vi "MC_10_19a_JW1.vi"() -> ()   [LabVIEW 2011]
uses:
  <vilib>/Utility/file.llb/Read From Spreadsheet File (string).vi
  <vilib>/Utility/inputDevices.llb/keyboardAcquire.vi
  <vilib>/Utility/file.llb/Write To Spreadsheet File (string).vi
  <vilib>/regexp/Match Regular Expression.xnode
panel:
  out "Column":string
  out "Row":string
  out "Date Recorded":string="Date Recorded"
  out "Concentration Recorded":string
  out "Solvent Recorded":string
  out "Method Recorded":string
  in  "?":T1(tab)
  out "Material Recorded":string
  in  "Treatment Concentration (mM):":dbl
  in  "Surface Treatment:":string
  in  "# Drops:":dbl
  in  "Solution Temp (C):":dbl
  in  "Relative Humidity (%):":dbl
  in  "Room Temp (F):":dbl
  in  "Time (s):":dbl
  out "Accel (RPM/s):":dbl
  in  "RPM:":dbl
  in  "Wait Time (s):":dbl
  in  "Sample #:":dbl
  in  "Fabricator:":string
  in  "Data File":path
  out "Data Folder":path
  in  "Image Folder":path
  out "Image File":path
  in  "Ramp (s):":dbl
  out "Mobility":dbl format="%#_4e"
  out "Length":dbl
  out "Width":dbl
  out "Dielectric (d)":dbl
  out "XY Graph":cluster{dbl[], dbl[]}[](graph)
  in  "NumPts":dbl=5.0
  in  "Cancel Button":bool
  in  "Next Button":bool
  in  "Previous Button":bool
  in  "Up Button":bool
  in  "Down Button":bool
  out "Data Name":string
  in  "Save Changes?":bool
  in  "New Dielectric":dbl
  in  "New Length":dbl
  in  "New Width":dbl
  out "New Mobility":dbl format="%#_4e"
  in  "Slide":dbl(slide) step=1.0 scale=-14.3..84.0 scale format="%#_1p"
  in  "Blank Button":bool
  in  "Zoom":i16(slide)=-3 scale=-5.0..5.0
  out "Image Out 2":T2(plugin-control)
  out "Image Out":T2(plugin-control)
  in  "Magnification":u16(ring) items=["5x", "10x", "20x", "50x", "80x"]
  out "Total Width":dbl
  out "Distances":dbl[](array[numeric])
  in  "Undo Button":bool
  in  "Remove Button":bool
  out "Recorded Mobility":dbl format="%#_4e"
  out "Index 3":string
  out "Image Name":string
  in  "Export":bool
  out "Threshold V":dbl
  out "New Vt":dbl
  in  "Manual":bool
  out "XY Graph 2":cluster{dbl[], dbl[]}[](graph)
  in  "Next Button 2":bool
  in  "Previous Button 2":bool
  in  "Slide 2":dbl(slide) step=1.0 scale=-1.0..82.0 scale format="%#_1p"
  out "S.T.S.":dbl
  out "New S.T.S.":dbl
  in  "NumPts 2":dbl=5.0
  out "Vt recorded":dbl
  out "STS recorded":dbl
  out "On/Off":dbl format="%#_3e"
  in  "Save Changes? 2":bool
  in  "Save Changes? 3":bool
  out "Export \nHeaders":string[](array[string])
  out "Current\nRecord":string[](array[string])
  out "Full Database":string[][](array[string])
  out "String":string
  in  "No Image":path=path "C:/Program Files/Mega Awesome/Image Not Found.png"
  in  "Project":path=path "C:/Program Files/Mega Awesome/DeviceData.opj"
  out "Index 2":dbl
  out "Array 8":dbl[](array[numeric])
  out "Array 7":dbl[](array[numeric])
  out "ROI Descriptor out":T3 {"Contours"."Type" items=["No Selection", "Point", "Line", "Rectangle", "Oval", "Polygon", "Freehand Region", "Annulus", "Unused2", "Unused3", "Broken Line", "Freehand Line", "Rotated Rectangle"]}
  out "ROI Descriptor":T3 {"Contours"."Type" items=["No Selection", "Point", "Line", "Rectangle", "Oval", "Polygon", "Freehand Region", "Annulus", "Unused2", "Unused3", "Broken Line", "Freehand Line", "Rotated Rectangle"]}
  out "Numeric 3":dbl
  out "Array 6":dbl[][](array[numeric])
  out "Cluster":T4
  out "Array 5":dbl[](array[numeric])
  out "Array 4":dbl[](array[numeric])
  out "Array 3":dbl[](array[numeric])
  out "Numeric 2":dbl
  out "Numeric":dbl
  out "Array 2":dbl[](array[numeric])
  out "Array":dbl[](array[numeric])
  out "Index":dbl
  out "Table Control 2":string[][](table)
  out "Table Control":string[][](table)
  in  "Row Start":dbl=20.0
  # "Data Locations"
  # "Data Location"
  # "Image Location"
  # "Sample Properties"
  # "Recorded"
  # "Calculated"
  # "Re-Calculated"
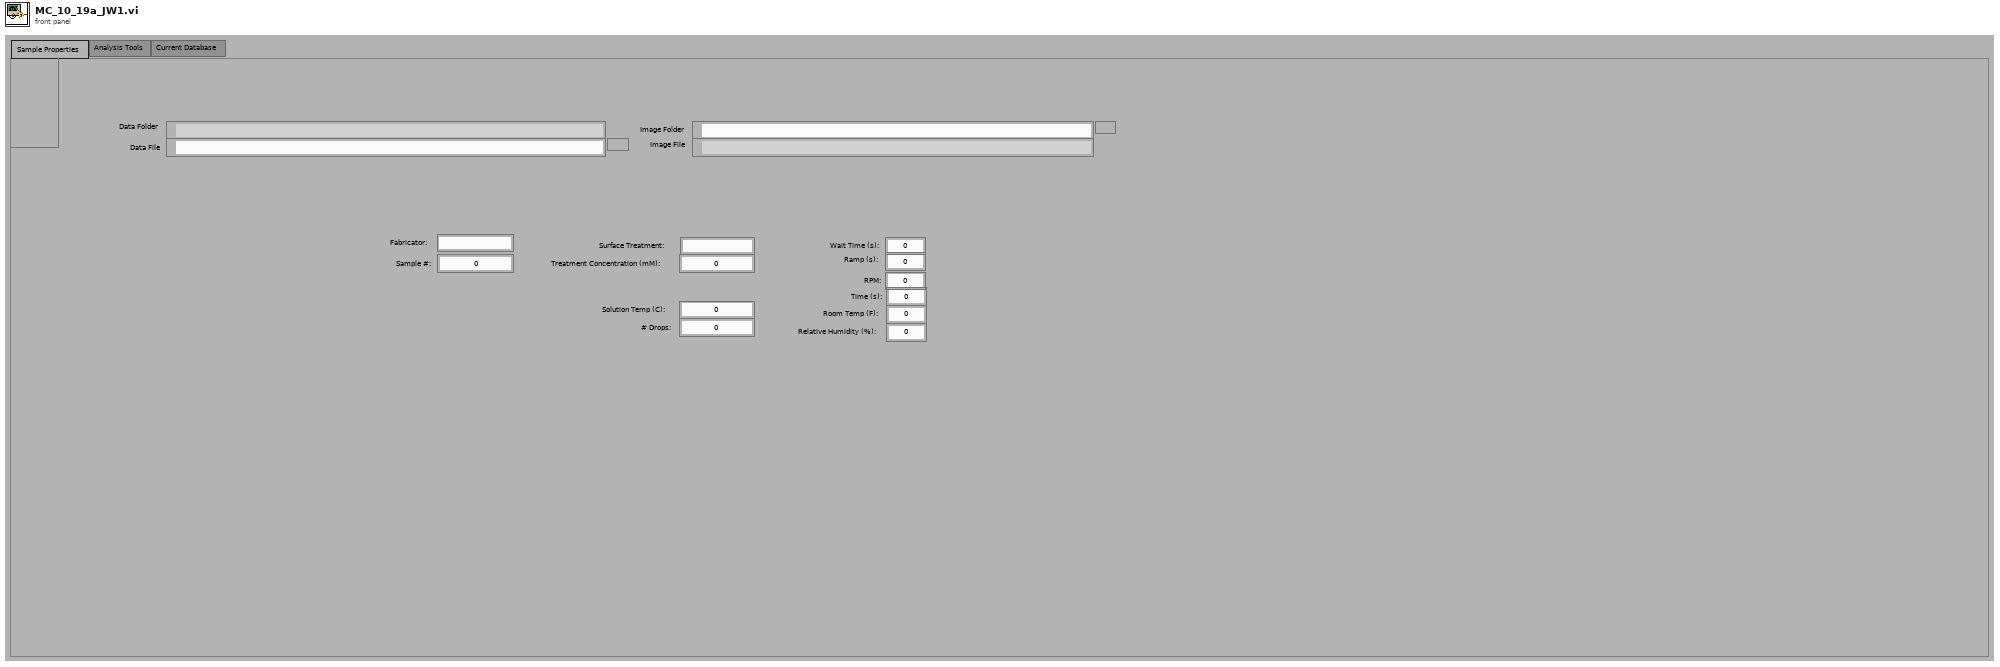
[diagram p1: front panel]
types:
  T1 = enum32{"Sample Properties", "Analysis Tools", "Current Database"}
  T2 = typedef "IMAQ Image.ctl" = refnum<image>
  T3 = typedef "ROI Descriptor" = cluster{"Global Rectangle":i32[], "Contours":cluster{"ID":enum32{"External", "Internal"}, "Type":u32, "Coordinates":i32[]}[]}
  T4 = cluster{"Numeric":dbl, "Numeric 2":dbl, "Numeric 3":dbl, "Numeric 4":dbl}
  T5 = cluster{"[0]":cluster{dbl[], dbl[]}, "[1]":cluster{dbl[], dbl[]}, "[2]":cluster{dbl[], dbl[]}, "[3]":cluster{dbl[], dbl[]}, "[4]":cluster{dbl[], dbl[]}, "[5]":cluster{dbl[], dbl[]}, "[6]":cluster{dbl[], dbl[]}, "[7]":cluster{dbl[], dbl[]}, "[8]":cluster{dbl[], dbl[]}}
  T6 = cluster{"Vt":dbl, "STS":dbl, "On/Off":dbl, "Deposition":string, "Solvent":string, "Concentration":string, "Material":string}
  T7 = cluster{"Global Rectangle":i32[], "Contours":cluster{"Contour Type":u32, "ROI Type":u32, "Points":i32[]}[]}
  T8 = typedef "LVBoundsTypeDef.ctl" = cluster{"Width":u32, "Height":u32}
  T9 = cluster{"Contour Type":u32, "ROI Type":u32, "Points":i32[]}[]
  T10 = enum16{"0", "1", "2", "3", "4", "5", "6", "7", "8", "9", "A", "B", "C", "D", "E", "F", "G", "H", "I", "J", "K", "L", "M", "N", "O", "P", "Q", "R", "S", "T", "U", "V", "W", "X", "Y", "Z", "F1", "F2", "F3", "F4", "F5", "F6", "F7", "F8", "F9", "F10", "F11", "F12", "F13", "F14", "F15", "ADD", "BACK", "BACKSLASH", "CAPITAL", "COMMA", "DECIMAL", "DELETE", "DIVIDE", "DOWN", "END", "EQUALS", "ESCAPE", "GRAVE (`)", "HOME", "INSERT", "LBRACKET", "LCONTROL", "LEFT", "L ALT", "LSHIFT", "LWIN", "MINUS", "MULTIPLY", "NEXT", "NUMLOCK", "NUMPAD_0", "NUMPAD_1", "NUMPAD_2", "NUMPAD_3", "NUMPAD_4", "NUMPAD_5", "NUMPAD_6", "NUMPAD_7", "NUMPAD_8", "NUMPAD_9", "PAUSE", "PERIOD", "PRIOR (PG UP)", "RBRACKET", "RCONTROL", "RETURN", "RIGHT", "R ALT", "RSHIFT", "RWIN", "SCROLL", "SEMICOLON", "SLASH", "SPACE", "SUBTRACT", "TAB", "UP", "ENTER (num pad)", "' (quote)"}[]
  T11 = cluster{i32[], cluster{"Contour Type":u32, "ROI Type":u32, "Points":i32[]}[]}
  T12 = enum16{"0", "1", "2", "3", "4", "5", "6", "7", "8", "9", "A", "B", "C", "D", "E", "F", "G", "H", "I", "J", "K", "L", "M", "N", "O", "P", "Q", "R", "S", "T", "U", "V", "W", "X", "Y", "Z", "F1", "F2", "F3", "F4", "F5", "F6", "F7", "F8", "F9", "F10", "F11", "F12", "F13", "F14", "F15", "ADD", "BACK", "BACKSLASH", "CAPITAL", "COMMA", "DECIMAL", "DELETE", "DIVIDE", "DOWN", "END", "EQUALS", "ESCAPE", "GRAVE (`)", "HOME", "INSERT", "LBRACKET", "LCONTROL", "LEFT", "L ALT", "LSHIFT", "LWIN", "MINUS", "MULTIPLY", "NEXT", "NUMLOCK", "NUMPAD_0", "NUMPAD_1", "NUMPAD_2", "NUMPAD_3", "NUMPAD_4", "NUMPAD_5", "NUMPAD_6", "NUMPAD_7", "NUMPAD_8", "NUMPAD_9", "PAUSE", "PERIOD", "PRIOR (PG UP)", "RBRACKET", "RCONTROL", "RETURN", "RIGHT", "R ALT", "RSHIFT", "RWIN", "SCROLL", "SEMICOLON", "SLASH", "SPACE", "SUBTRACT", "TAB", "UP", "ENTER (num pad)", "' (quote)"}
  T13 = cluster{string, sgl, bool, bool, bool, bool, bool, bool, i32}
  T14 = cluster{i32, cluster{string, sgl, bool, bool, bool, bool, bool, bool, i32}, i32, i32}
  T15 = cluster{"Contour Type":u32, "ROI Type":u32, "Points":i32[]}
  T16 = cluster{"Points[0]":i32, "Points[1]":i32, "Points[2]":i32, "Points[3]":i32, "Points[4]":i32, "Points[5]":i32, "Points[6]":i32, "Points[7]":i32, "Points[8]":i32}
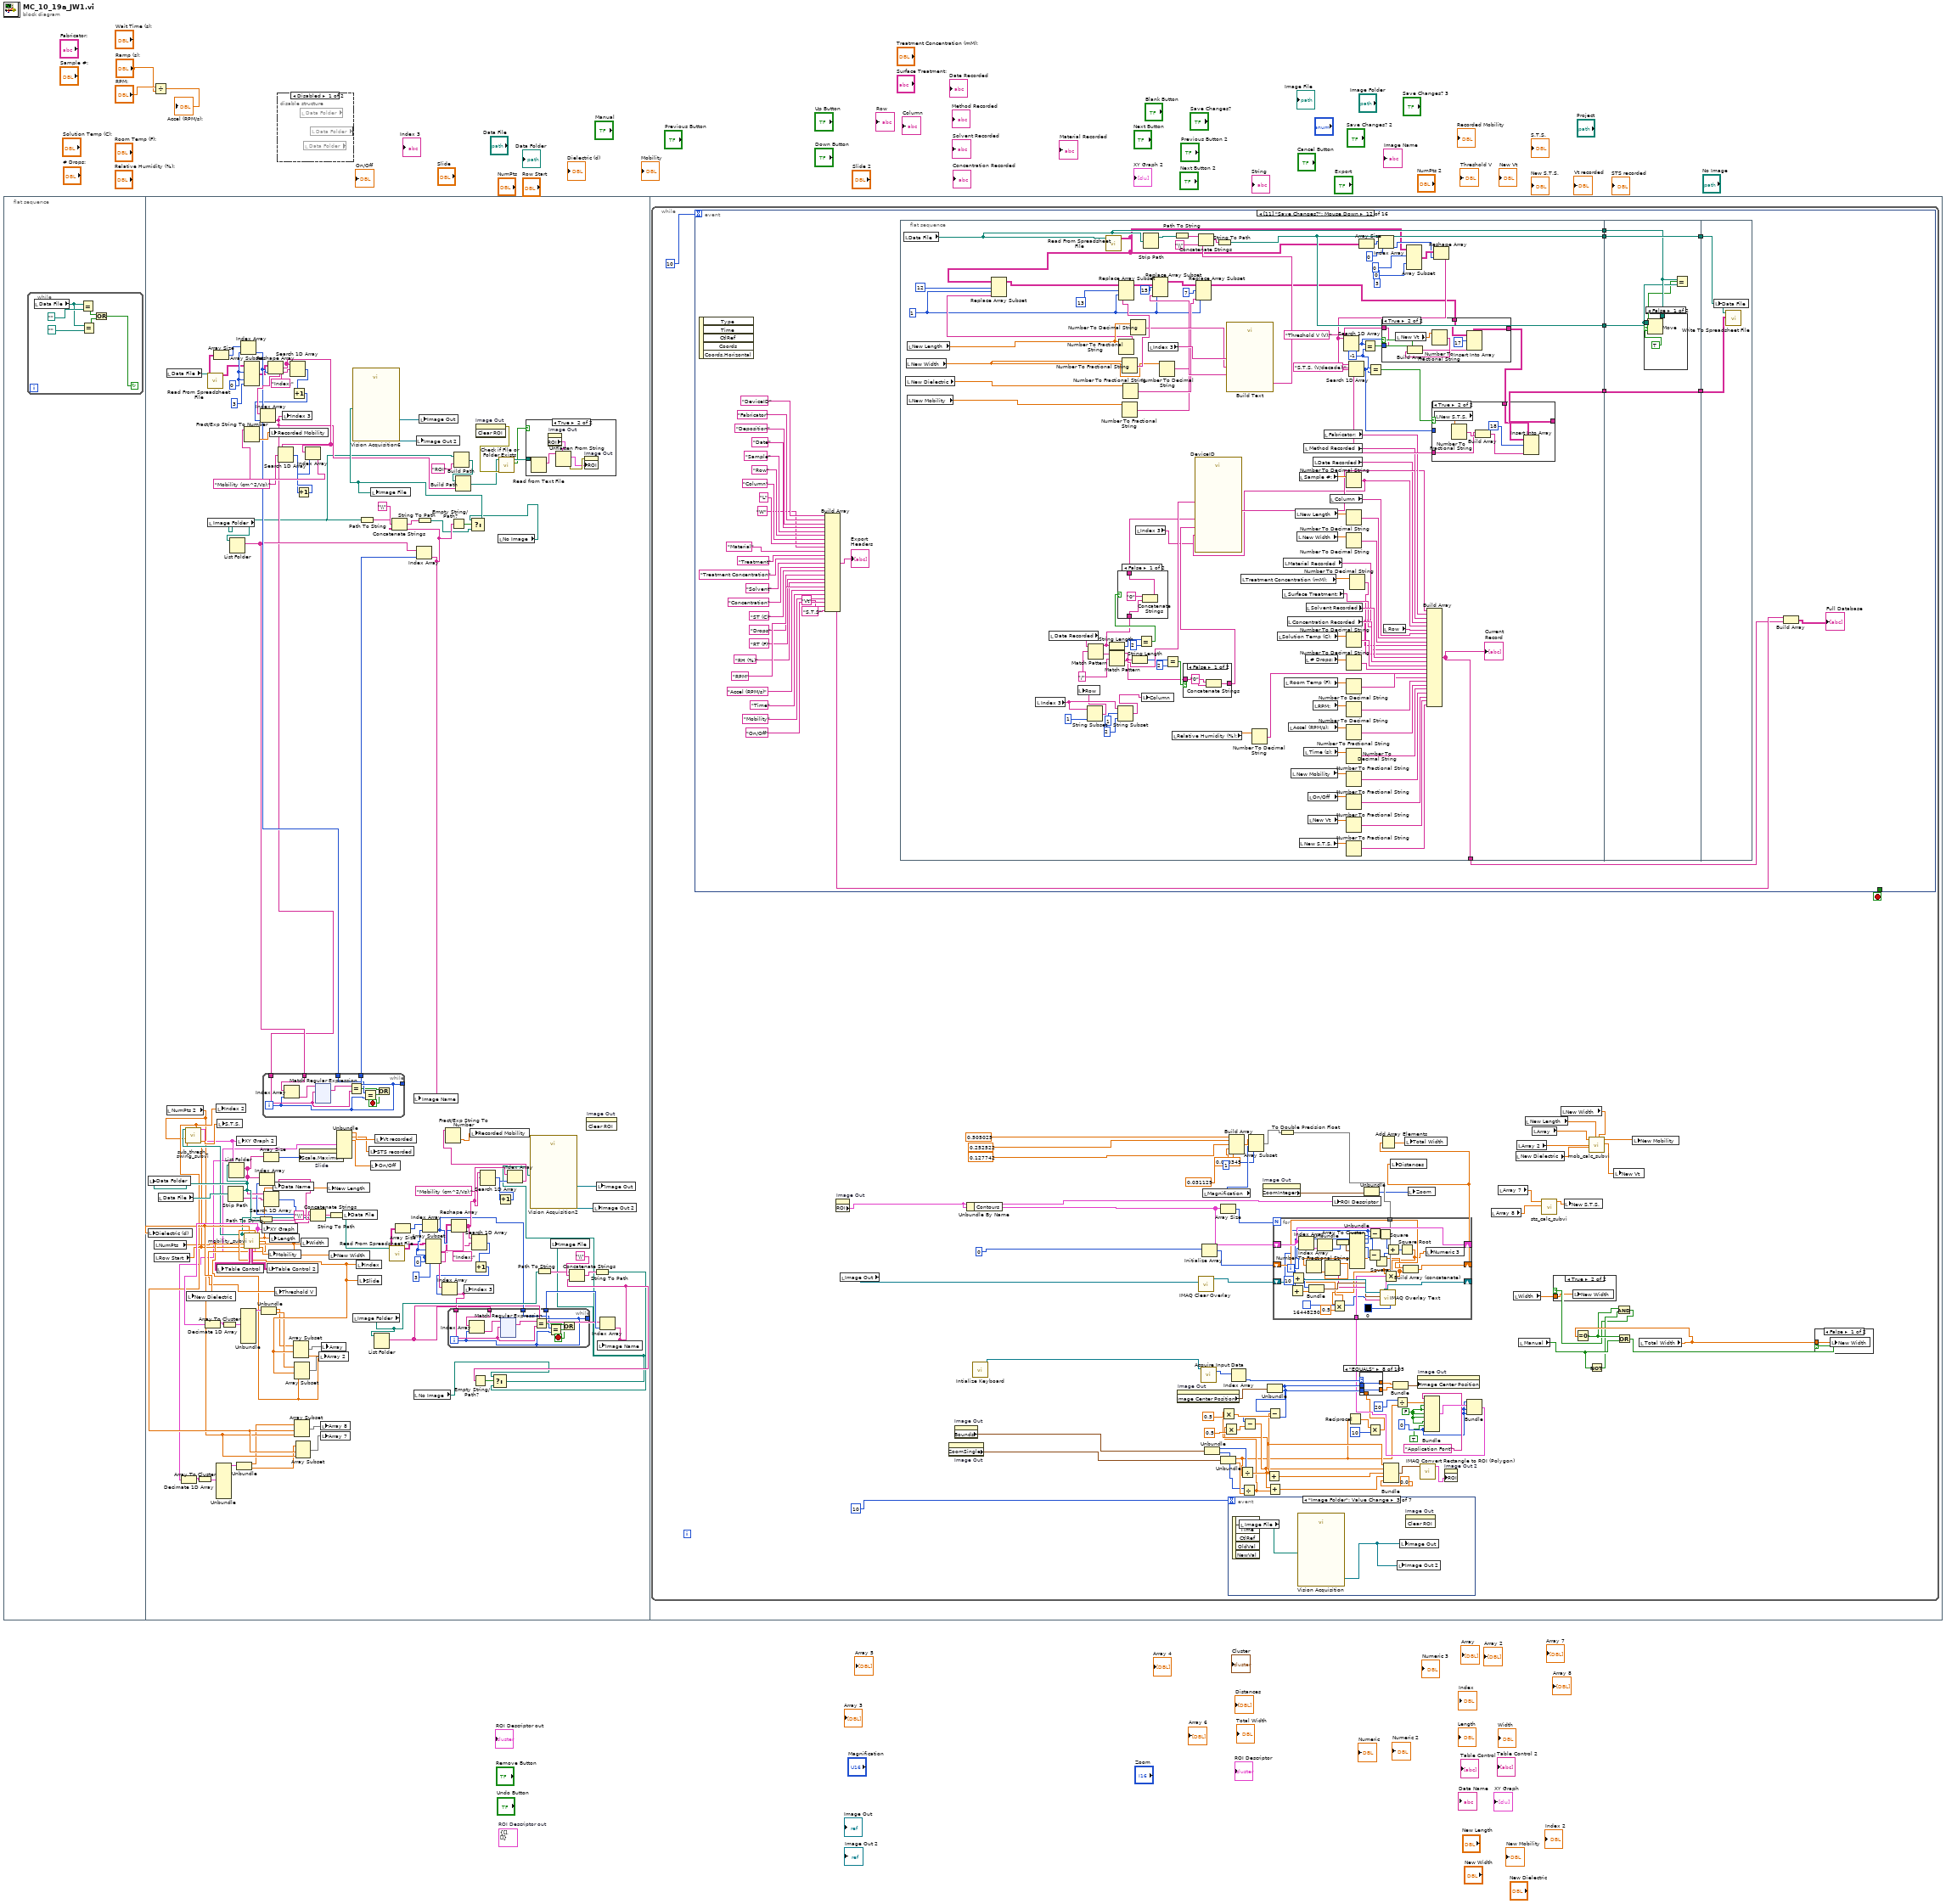
[diagram p0: block diagram]
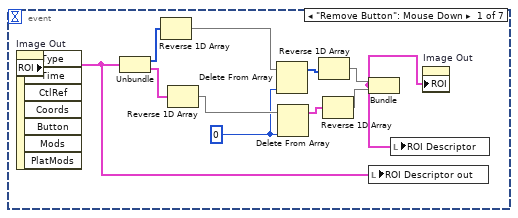
[diagram p5: hidden frame]
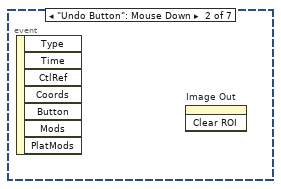
[diagram p6: hidden frame]
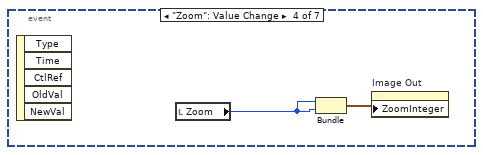
[diagram p7: hidden frame]
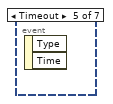
[diagram p8: hidden frame]
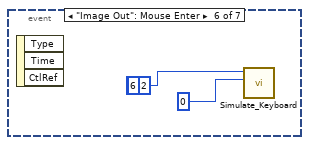
[diagram p9: hidden frame]
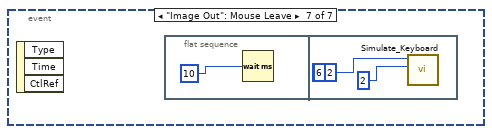
[diagram p10: hidden frame]
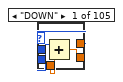
[diagram p11: hidden frame]
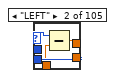
[diagram p12: hidden frame]
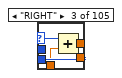
[diagram p13: hidden frame]
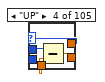
[diagram p14: hidden frame]
diagram:
  (unwired) T3 {"Global Rectangle"=[], "Contours"=[]}  # ROI Descriptor out
  n1 = flat-sequence {
    frame #0 {
      n2 = while {
        stop <- w4 continue-if-true
        n3 = local read "Data File"() -> (w6:path)
        n4 = Equal?(x=w6, y=path "") -> (x = y?=w8:bool)
        n5 = Equal?(x=w6, y=path "") -> (x = y?=w7:bool)
        n6 = Or(x=w8, y=w7) -> (x .or. y?=w4:bool)
      }
    }
    frame #1 {
      w70 = 0
      w100 = 0
      n7 = local read "NumPts"() -> (w45:dbl)
      n8 = local read "Row Start"() -> (w44:dbl)
      n9 = local read "Data File"() -> (w74:path)
      n10 = local read "Data File"() -> (w95:path)
      n11 = local read "NumPts 2"() -> (w39:dbl)
      n12 = call-poly <vilib>:"Read From Spreadsheet File.vi"("file path (dialog if empty)"=w95) -> ("all rows"=w98:string[][])  [unwired: 6 in, 4 out]
      n13 = local read "Image Folder"() -> (w10:path)
      n14 = Array Size(array=w98) -> (size(s)=w99:i32[])
      n15 = Strip Path(path=w74) -> (stripped path=w75:path, name=w56:string)
      n16 = local write "Data Folder"(w75) -> ()
      n17 = List Folder(path=w75) -> (filenames=w64:string[])  [unwired: 3 in, 3 out]
      n18 = List Folder(path=w10) -> (filenames=w104:string[])  [unwired: 3 in, 3 out]
      n19 = Index Array(array=w99, index=w100) -> (element=w106:i32)
      n20 = Array Subset(array=w98, index (row)=w100, index (col)=w100, length (col)=3) -> (w97:string[][])  [unwired: 1 in]
      n21 = Path To String(path=w75) -> (string=w55:string)
      n22 = Array Size(array=w64) -> (size(s)=w65:i32)
      n23 = Search 1D Array(1D array=w64, element=w56) -> (index of element=w63:i32)  [unwired: 1 in]
      n24 = Index Array(array=w64, index=w63) -> (element=w62:string)
      n25 = Reshape Array(w97, w106) -> (w116:string[])
      n26 = local write "Data Name"(w62) -> ()
      n27 = Search 1D Array(1D array=w116, element="Mobility (cm^2/Vs):") -> (index of element=w111:i32)  [unwired: 1 in]
      n28 = Search 1D Array(1D array=w116, element="Index:") -> (index of element=w103:i32)  [unwired: 1 in]
      n29 = Increment(x=w103) -> (x+1=w102:i32)
      n30 = Index Array(array=w116, index=w102) -> (element=w11:string)
      n31 = while {
        tunnel: w104 -> [w249]
        tunnel: w11 -> [w247]
        tunnel: [w246] -> _
        tunnel: [w246] -> w105
        tunnel: w106 -> [w245]
        i -> [w246]
        stop <- w242 stop-if-true
        n32 = Index Array(array=w249, index=w246) -> (element=w250:string)
        n33 = xnode "Match Regular Expression"("input string"=w250, "regular expression"=w247) -> ("whole match"=w248:string)  [unwired: 4 in, 4 out]
        n34 = Equal?(x=w248, y=w247) -> (x = y?=w244:bool)
        n35 = Equal?(x=w245, y=w246) -> (x = y?=w243:bool)
        n36 = Or(x=w244, y=w243) -> (x .or. y?=w242:bool)
      }
      n37 = local write "Index 3"(w11) -> ()
      n38 = Increment(x=w111) -> (x+1=w112:i32)
      n39 = property on="Slide" class="Slide (strict)"("Scale.Maximum"=w65) -> ()  [unwired: 2 in, 2 out]
      n40 = Index Array(array=w116, index=w112) -> (element=w114:string)
      n41 = Fract/Exp String To Number(string=w114) -> (number=w115:dbl)  [unwired: 3 in, 1 out]
      n42 = local write "Recorded Mobility"(w115) -> ()
      n43 = Concatenate Strings(w55, "\\", w62) -> (w57:string)
      n44 = String To Path(string=w57) -> (path=w46:path)
      n45 = call "sub_thresh_swing_subvi.vi"("Path"=w46, "NumPts"=w39, "Row Start"=w44) -> ("Index"=w40:dbl, "XY Graph"=w35:cluster{dbl[], dbl[]}[], "Sub Threshold Swing"=w47:dbl)  [unwired: 8 in, 2 out]
      n46 = Decimate 1D Array(w35) -> (w36:cluster{dbl[], dbl[]}[])  [unwired: 1 out]
      n47 = Array To Cluster(array=w36) -> (cluster=w38:T5)
      n48 = local write "Index 2"(w40) -> ()
      n49 = Unbundle(w38) -> ("[0]"=w37:cluster{dbl[], dbl[]})  [unwired: 8 out]
      n50 = local write "S.T.S."(w47) -> ()
      n51 = local write "XY Graph 2"(w35) -> ()
      n52 = Unbundle(w37) -> (w33:dbl[], w32:dbl[])
      n53 = call "mobility_subvi.vi"("Path"=w46, "NumPts"=w45, "Row Start"=w44) -> ("Dielectric (d)"=w51:dbl, "Index"=w52:dbl, "XY Graph"=w94:cluster{dbl[], dbl[]}[], "Length"=w50:dbl, "Vt"=w48:dbl, "Width"=w49:dbl, "Table Control"=w59:string[][], "Table Control 2"=w60:string[][], "Recorded"=w29:T6, "Mobility"=w61:dbl)  [unwired: 2 in, 1 out]
      n54 = local write "Dielectric (d)"(w51) -> ()
      n55 = local write "New Dielectric"(w51) -> ()
      n56 = Decimate 1D Array(w94) -> (w93:cluster{dbl[], dbl[]}[])  [unwired: 1 out]
      n57 = local write "Table Control"(w59) -> ()
      n58 = Array To Cluster(array=w93) -> (cluster=w91:T5)
      n59 = Unbundle(w91) -> ("[0]"=w92:cluster{dbl[], dbl[]})  [unwired: 8 out]
      n60 = Unbundle(w92) -> (w34:dbl[], w41:dbl[])
      n61 = local write "XY Graph"(w94) -> ()
      n62 = local write "Table Control 2"(w60) -> ()
      n63 = local write "Mobility"(w61) -> ()
      n64 = local write "Length"(w50) -> ()
      n65 = local write "Threshold V"(w48) -> ()
      n66 = Array Subset(array=w34, index=w52, length=w45) -> (w53:dbl[])
      n67 = Array Subset(array=w41, index=w52, length=w45) -> (w54:dbl[])
      n68 = Array Subset(array=w33, index=w40, length=w39) -> (w43:dbl[])
      n69 = Array Subset(array=w32, index=w40, length=w39) -> (w42:dbl[])
      n70 = local write "Width"(w49) -> ()
      n71 = local write "Array 2"(w54) -> ()
      n72 = local write "Array 8"(w43) -> ()
      n73 = local write "Array 7"(w42) -> ()
      n74 = local write "Array"(w53) -> ()
      n75 = local write "New Length"(w50) -> ()
      n76 = local write "New Width"(w49) -> ()
      n77 = Unbundle(w29) -> ("Vt"=w31:dbl, "STS"=w30:dbl, "On/Off"=w28:dbl)  [unwired: 4 out]
      n78 = local write "Data File"(w46) -> ()
      n79 = local read "Image Folder"() -> (w81:path)
      n80 = local write "Index"(w52) -> ()
      n81 = local write "Slide"(w52) -> ()
      n82 = Path To String(path=w10) -> (string=w108:string)
      n83 = local write "STS recorded"(w30) -> ()
      n84 = local write "On/Off"(w28) -> ()
      n85 = List Folder(path=w81) -> (filenames=w77:string[])  [unwired: 3 in, 3 out]
      n86 = local write "Vt recorded"(w31) -> ()
      n87 = call-poly <vilib>:"Read From Spreadsheet File.vi"("file path (dialog if empty)"=w46) -> ("all rows"=w68:string[][])  [unwired: 6 in, 4 out]
      n88 = Array Size(array=w68) -> (size(s)=w69:i32[])
      n89 = local read "No Image"() -> (w19:path)
      n90 = Index Array(array=w104, index=w105) -> (element=w27:string)
      n91 = Concatenate Strings(w108, "\\", w27) -> (w109:string)
      n92 = local write "Image Name"(w27) -> ()
      n93 = String To Path(string=w109) -> (path=w25:path)
      n94 = Index Array(array=w69, index=w70) -> (element=w80:i32)
      n95 = Array Subset(array=w68, index (row)=w70, index (col)=w70, length (col)=3) -> (w67:string[][])  [unwired: 1 in]
      n96 = Empty String/Path?(string/path=w27) -> (empty?=w26:bool)
      n97 = Reshape Array(w67, w80) -> (w90:string[])
      n98 = Build Path(base path=w10, name or relative path="ROI") -> (appended path=w13:path)
      n99 = Build Path(base path=w13, name or relative path=w11) -> (appended path=w12:path)
      n100 = Search 1D Array(1D array=w90, element="Index:") -> (index of element=w73:i32)  [unwired: 1 in]
      n101 = Increment(x=w73) -> (x+1=w72:i32)
      n102 = Index Array(array=w90, index=w72) -> (element=w78:string)
      n103 = while {
        tunnel: w77 -> [w129]
        tunnel: w78 -> [w127]
        tunnel: [w126] -> _
        tunnel: [w126] -> w79
        tunnel: w80 -> [w125]
        i -> [w126]
        stop <- w122 stop-if-true
        n104 = Index Array(array=w129, index=w126) -> (element=w130:string)
        n105 = xnode "Match Regular Expression"("input string"=w130, "regular expression"=w127) -> ("whole match"=w128:string)  [unwired: 4 in, 4 out]
        n106 = Equal?(x=w128, y=w127) -> (x = y?=w124:bool)
        n107 = Equal?(x=w125, y=w126) -> (x = y?=w123:bool)
        n108 = Or(x=w124, y=w123) -> (x .or. y?=w122:bool)
      }
      n109 = local write "Index 3"(w78) -> ()
      n110 = invoke on="Image Out" class="ImageControl" method="Clear ROI"() -> (error out=w17:errorcluster)  [unwired: 3 in, 2 out]
      n111 = Search 1D Array(1D array=w90, element="Mobility (cm^2/Vs):") -> (index of element=w85:i32)  [unwired: 1 in]
      n112 = local read "No Image"() -> (w18:path)
      n113 = Select(t=w18, s=w26, f=w25) -> (s? t:f=w24:path)
      n114 = call "Vision Acquisition6"("Image Path"=w24) -> ("Image Out"=w107:T2)  [unwired: 25 in, 1 out]
      n115 = local write "Image File"(w24) -> ()
      n116 = local write "Image Out 2"(w107) -> ()
      n117 = local write "Image Out"(w107) -> ()
      n118 = Increment(x=w85) -> (x+1=w86:i32)
      n119 = call <vilib>:"Check if File or Folder Exists.vi"("error in (no error)"=w17, "path"=w12) -> ("file or folder exists?"=w15:bool, "dup path"=w16:path)  [unwired: 7 in, 1 out]
      n120 = Index Array(array=w90, index=w86) -> (element=w88:string)
      n121 = Fract/Exp String To Number(string=w88) -> (number=w89:dbl)  [unwired: 3 in, 1 out]
      n122 = local write "Recorded Mobility"(w89) -> ()
      n123 = case shown="True" w15 {
        tunnel: w16 -> [_ w117]
        frame False {
        }
        frame True {
          n124 = Read from Text File(file (use dialog)=w117) -> (text=w121:string)  [unwired: 3 in, 3 out]
          n125 = property on="Image Out" class="ImageControl"() -> ("ROI"=w118:T7)  [unwired: 2 in, 2 out]
          n126 = Unflatten From String(type=w118, binary string=w121) -> (value=w119:T7, error out=w120:errorcluster)  [unwired: 3 in, 1 out]
          n127 = property on="Image Out" class="ImageControl"(error in=w120, "ROI"=w119) -> ()  [unwired: 1 in, 2 out]
        }
      }
      n128 = Path To String(path=w81) -> (string=w82:string)
      n129 = invoke on="Image Out" class="ImageControl" method="Clear ROI"() -> ()  [unwired: 3 in, 3 out]
      n130 = Index Array(array=w77, index=w79) -> (element=w22:string)
      n131 = Empty String/Path?(string/path=w22) -> (empty?=w23:bool)
      n132 = Concatenate Strings(w82, "\\", w22) -> (w83:string)
      n133 = String To Path(string=w83) -> (path=w21:path)
      n134 = Select(t=w19, s=w23, f=w21) -> (s? t:f=w20:path)
      n135 = call "Vision Acquisition2"("Image Path"=w20) -> ("Image Out"=w76:T2)  [unwired: 25 in, 1 out]
      n136 = local write "Image File"(w20) -> ()
      n137 = local write "Image Out 2"(w76) -> ()
      n138 = local write "Image Out"(w76) -> ()
      n139 = local write "Image Name"(w22) -> ()
    }
    frame #2 {
      n140 = while {
        stop <- w441 stop-if-true
        w391 = FALSE
        w389 = 0
        n141 = event shown="[11] \"Save Changes?\": Mouse Down" {
          selector: _ -> [_ _ _ _ _ _ _ _ _ _ _ _ _ _ _ _]
          dyn-events: _ -> [_ _ _ _ _ _ _ _ _ _ _ _ _ _ _ _]
          timeout: 10 -> [_ _ _ _ _ _ _ _ _ _ _ _ _ _ _ _]
          tunnel: [_ _ _ _ _ _ _ _ _ _ _ _ _ TRUE _ TRUE] -> w441
          event Timeout {
            n142 = event-data() -> ()  [unwired: 1 in, 2 out]
          }
          event "Down Button": Mouse Down {
            w789 = 0
            n143 = event-data() -> ()  [unwired: 1 in, 7 out]
            n144 = local read "NumPts 2"() -> (w750:dbl)
            n145 = local read "NumPts"() -> (w757:dbl)
            n146 = local read "Row Start"() -> (w756:dbl)
            n147 = local read "Data File"() -> (w794:path)
            n148 = property on="Image Out" class="ImageControl"() -> (error out=w719:errorcluster, "Image Center Position"=w723:cluster{"X":u32, "Y":u32})  [unwired: 2 in, 1 out]
            n149 = Unbundle(w723) -> ("X"=w721:u32)  [unwired: 1 out]
            n150 = Strip Path(path=w794) -> (stripped path=w785:path, name=w807:string)
            n151 = local write "Data Folder"(w785) -> ()
            n152 = List Folder(path=w785) -> (filenames=w800:string[], error out=w728:errorcluster)  [unwired: 3 in, 2 out]
            n153 = Array Size(array=w800) -> (size(s)=w795:i32)
            n154 = Bundle("X"=w721, 0) -> (w722:cluster{"X":u32, i32})  [unwired: 1 in]
            n155 = Path To String(path=w785) -> (string=w808:string)
            n156 = Search 1D Array(1D array=w800, element=w807) -> (index of element=w797:i32)  [unwired: 1 in]
            n157 = property on="Image Out" class="ImageControl"(error in=w719, "Image Center Position"=w722) -> ()  [unwired: 1 in, 2 out]
            n158 = Decrement(x=w795) -> (x-1=w798:i32)
            n159 = Equal?(x=w797, y=w798) -> (x = y?=w799:bool)
            n160 = case shown="False" w799 {
              tunnel: w797 -> [w935 _]
              tunnel: [w934 0] -> w796
              frame False {
                n161 = Increment(x=w935) -> (x+1=w934:i32)
              }
              frame True {
              }
            }
            n162 = Index Array(array=w800, index=w796) -> (element=w801:string)
            n163 = local write "Data Name"(w801) -> ()
            n164 = Concatenate Strings(w808, "\\", w801) -> (w806:string)
            n165 = String To Path(string=w806) -> (path=w758:path)
            n166 = call "sub_thresh_swing_subvi.vi"("Path"=w758, "NumPts"=w750, "Row Start"=w756) -> ("Index"=w751:dbl, "XY Graph"=w746:cluster{dbl[], dbl[]}[], "Sub Threshold Swing"=w759:dbl)  [unwired: 8 in, 2 out]
            n167 = Decimate 1D Array(w746) -> (w749:cluster{dbl[], dbl[]}[])  [unwired: 1 out]
            n168 = Array To Cluster(array=w749) -> (cluster=w747:T5)
            n169 = Unbundle(w747) -> ("[0]"=w748:cluster{dbl[], dbl[]})  [unwired: 8 out]
            n170 = Unbundle(w748) -> (w745:dbl[], w744:dbl[])
            n171 = local write "S.T.S."(w759) -> ()
            n172 = local write "XY Graph 2"(w746) -> ()
            n173 = local write "Index 2"(w751) -> ()
            n174 = call "mobility_subvi.vi"("Path"=w758, "NumPts"=w757, "Row Start"=w756) -> ("Dielectric (d)"=w761:dbl, "Date Created"=w718:string, "Index"=w766:dbl, "XY Graph"=w769:cluster{dbl[], dbl[]}[], "Length"=w760:dbl, "Vt"=w762:dbl, "Width"=w734:dbl, "Table Control"=w804:string[][], "Table Control 2"=w803:string[][], "Recorded"=w743:T6, "Mobility"=w802:dbl)  [unwired: 2 in]
            n175 = local write "Dielectric (d)"(w761) -> ()
            n176 = local write "Threshold V"(w762) -> ()
            n177 = local write "New Dielectric"(w761) -> ()
            n178 = Decimate 1D Array(w769) -> (w770:cluster{dbl[], dbl[]}[])  [unwired: 1 out]
            n179 = Array To Cluster(array=w770) -> (cluster=w772:T5)
            n180 = local write "Table Control"(w804) -> ()
            n181 = Unbundle(w772) -> ("[0]"=w771:cluster{dbl[], dbl[]})  [unwired: 8 out]
            n182 = Unbundle(w771) -> (w753:dbl[], w752:dbl[])
            n183 = local write "XY Graph"(w769) -> ()
            n184 = local write "Table Control 2"(w803) -> ()
            n185 = local write "Mobility"(w802) -> ()
            n186 = Array Subset(array=w753, index=w766, length=w757) -> (w768:dbl[])
            n187 = Array Subset(array=w752, index=w766, length=w757) -> (w767:dbl[])
            n188 = Unbundle(w743) -> ("Vt"=w742:dbl, "STS"=w741:dbl, "On/Off"=w740:dbl, "Deposition"=w717:string, "Solvent"=w716:string, "Concentration"=w715:string, "Material"=w714:string)
            n189 = local write "On/Off"(w740) -> ()
            n190 = local write "Width"(w734) -> ()
            n191 = local write "Length"(w760) -> ()
            n192 = local write "Array 2"(w767) -> ()
            n193 = local write "Array"(w768) -> ()
            n194 = local write "Slide"(w766) -> ()
            n195 = local write "Index"(w766) -> ()
            n196 = local write "STS recorded"(w741) -> ()
            n197 = local write "Date Recorded"(w718) -> ()
            n198 = local write "Solvent Recorded"(w716) -> ()
            n199 = local write "Concentration Recorded"(w715) -> ()
            n200 = local write "Method Recorded"(w717) -> ()
            n201 = local write "Vt recorded"(w742) -> ()
            n202 = Array Subset(array=w745, index=w751, length=w750) -> (w755:dbl[])
            n203 = Array Subset(array=w744, index=w751, length=w750) -> (w754:dbl[])
            n204 = local write "Material Recorded"(w714) -> ()
            n205 = local write "New Width"(w734) -> ()
            n206 = local write "Data File"(w758) -> ()
            n207 = local write "New Length"(w760) -> ()
            n208 = local write "Array 8"(w755) -> ()
            n209 = local write "Array 7"(w754) -> ()
            n210 = call-poly <vilib>:"Read From Spreadsheet File.vi"("file path (dialog if empty)"=w758) -> ("all rows"=w791:string[][])  [unwired: 6 in, 4 out]
            n211 = local read "Image Folder"() -> (w725:path)
            n212 = Array Size(array=w791) -> (size(s)=w790:i32[])
            n213 = List Folder(path=w725, error in=w728) -> (filenames=w784:string[], error out=w729:errorcluster)  [unwired: 2 in, 2 out]
            n214 = Index Array(array=w790, index=w789) -> (element=w764:i32)
            n215 = Subtract(x=w764, y=20) -> (x-y=w763:i32)
            n216 = property on="Slide" class="Slide (strict)"("Scale.Maximum"=w763) -> ()  [unwired: 2 in, 2 out]
            n217 = Array Subset(array=w791, index (row)=w789, index (col)=w789, length (col)=3) -> (w792:string[][])  [unwired: 1 in]
            n218 = Reshape Array(w792, w764) -> (w773:string[])
            n219 = local read "No Image"() -> (w735:path)
            n220 = Search 1D Array(1D array=w773, element="Mobility (cm^2/Vs):") -> (index of element=w778:i32)  [unwired: 1 in]
            n221 = Search 1D Array(1D array=w773, element="Index:") -> (index of element=w786:i32)  [unwired: 1 in]
            n222 = Increment(x=w786) -> (x+1=w787:i32)
            n223 = Index Array(array=w773, index=w787) -> (element=w727:string)
            n224 = while {
              tunnel: w784 -> [w821]
              tunnel: w727 -> [w819]
              tunnel: [w818] -> _
              tunnel: [w818] -> w783
              tunnel: w764 -> [w817]
              i -> [w818]
              stop <- w814 stop-if-true
              n225 = Index Array(array=w821, index=w818) -> (element=w822:string)
              n226 = xnode "Match Regular Expression"("input string"=w822, "regular expression"=w819) -> ("whole match"=w820:string)  [unwired: 4 in, 4 out]
              n227 = Equal?(x=w820, y=w819) -> (x = y?=w816:bool)
              n228 = Equal?(x=w817, y=w818) -> (x = y?=w815:bool)
              n229 = Or(x=w816, y=w815) -> (x .or. y?=w814:bool)
            }
            n230 = local write "Index 3"(w727) -> ()
            n231 = Increment(x=w778) -> (x+1=w777:i32)
            n232 = Build Path(base path=w725, name or relative path="ROI") -> (appended path=w724:path)
            n233 = Index Array(array=w773, index=w777) -> (element=w775:string)
            n234 = Fract/Exp String To Number(string=w775) -> (number=w774:dbl)  [unwired: 3 in, 1 out]
            n235 = local write "Recorded Mobility"(w774) -> ()
            n236 = Build Path(base path=w724, name or relative path=w727) -> (appended path=w733:path)
            n237 = Path To String(path=w725) -> (string=w781:string)
            n238 = invoke on="Image Out" class="ImageControl" method="Clear ROI"(error in=w729) -> (error out=w732:errorcluster)  [unwired: 2 in, 2 out]
            n239 = call <vilib>:"Check if File or Folder Exists.vi"("error in (no error)"=w732, "path"=w733) -> ("file or folder exists?"=w730:bool, "dup path"=w731:path)  [unwired: 7 in, 1 out]
            n240 = Index Array(array=w784, index=w783) -> (element=w738:string)
            n241 = Empty String/Path?(string/path=w738) -> (empty?=w739:bool)
            n242 = Concatenate Strings(w781, "\\", w738) -> (w780:string)
            n243 = String To Path(string=w780) -> (path=w737:path)
            n244 = Select(t=w735, s=w739, f=w737) -> (s? t:f=w736:path)
            n245 = call "Vision Acquisition4"("Image Path"=w736) -> ("Image Out"=w782:T2)  [unwired: 25 in, 1 out]
            n246 = local write "Image File"(w736) -> ()
            n247 = local write "Image Name"(w738) -> ()
            n248 = local write "Image Out 2"(w782) -> ()
            n249 = local write "Image Out"(w782) -> ()
            n250 = invoke on="Image Out" class="ImageControl" method="Clear ROI"() -> ()  [unwired: 3 in, 3 out]
            n251 = case shown="True" w730 {
              tunnel: w731 -> [_ w809]
              frame False {
              }
              frame True {
                n252 = Read from Text File(file (use dialog)=w809) -> (text=w813:string)  [unwired: 3 in, 3 out]
                n253 = property on="Image Out" class="ImageControl"() -> ("ROI"=w810:T7)  [unwired: 2 in, 2 out]
                n254 = Unflatten From String(type=w810, binary string=w813) -> (value=w811:T7, error out=w812:errorcluster)  [unwired: 3 in, 1 out]
                n255 = property on="Image Out" class="ImageControl"(error in=w812, "ROI"=w811) -> ()  [unwired: 1 in, 2 out]
              }
            }
          }
          event "Data File": Value Change {
            w1008 = 0
            n256 = event-data() -> ()  [unwired: 1 in, 5 out]
            n257 = local read "NumPts"() -> (w976:dbl)
            n258 = local read "Row Start"() -> (w975:dbl)
            n259 = local read "Data File"() -> (w1004:path)
            n260 = local read "NumPts 2"() -> (w969:dbl)
            n261 = property on="Image Out" class="ImageControl"() -> (error out=w937:errorcluster, "Image Center Position"=w941:cluster{"X":u32, "Y":u32})  [unwired: 2 in, 1 out]
            n262 = Strip Path(path=w1004) -> (stripped path=w1003:path, name=w1021:string)
            n263 = local write "Data Folder"(w1003) -> ()
            n264 = List Folder(path=w1003) -> (filenames=w1013:string[], error out=w947:errorcluster)  [unwired: 3 in, 2 out]
            n265 = Unbundle(w941) -> ("X"=w939:u32)  [unwired: 1 out]
            n266 = Path To String(path=w1003) -> (string=w1022:string)
            n267 = Search 1D Array(1D array=w1013, element=w1021) -> (index of element=w1014:i32)  [unwired: 1 in]
            n268 = Index Array(array=w1013, index=w1014) -> (element=w1015:string)
            n269 = Bundle("X"=w939, 0) -> (w940:cluster{"X":u32, i32})  [unwired: 1 in]
            n270 = local write "Data Name"(w1015) -> ()
            n271 = property on="Image Out" class="ImageControl"(error in=w937, "Image Center Position"=w940) -> ()  [unwired: 1 in, 2 out]
            n272 = Concatenate Strings(w1022, "\\", w1015) -> (w1020:string)
            n273 = String To Path(string=w1020) -> (path=w977:path)
            n274 = call "sub_thresh_swing_subvi.vi"("Path"=w977, "NumPts"=w969, "Row Start"=w975) -> ("Index"=w970:dbl, "XY Graph"=w965:cluster{dbl[], dbl[]}[], "Sub Threshold Swing"=w974:dbl)  [unwired: 8 in, 2 out]
            n275 = Decimate 1D Array(w965) -> (w968:cluster{dbl[], dbl[]}[])  [unwired: 1 out]
            n276 = Array To Cluster(array=w968) -> (cluster=w966:T5)
            n277 = Unbundle(w966) -> ("[0]"=w967:cluster{dbl[], dbl[]})  [unwired: 8 out]
            n278 = Unbundle(w967) -> (w963:dbl[], w962:dbl[])
            n279 = local write "Index 2"(w970) -> ()
            n280 = call "mobility_subvi.vi"("Path"=w977, "NumPts"=w976, "Row Start"=w975) -> ("Dielectric (d)"=w979:dbl, "Index"=w984:dbl, "XY Graph"=w987:cluster{dbl[], dbl[]}[], "Length"=w978:dbl, "Vt"=w980:dbl, "Width"=w952:dbl, "Table Control"=w1018:string[][], "Table Control 2"=w1017:string[][], "Recorded"=w959:T6, "Mobility"=w1016:dbl)  [unwired: 2 in, 1 out]
            n281 = local write "Dielectric (d)"(w979) -> ()
            n282 = local write "New Dielectric"(w979) -> ()
            n283 = Decimate 1D Array(w987) -> (w988:cluster{dbl[], dbl[]}[])  [unwired: 1 out]
            n284 = local write "Table Control"(w1018) -> ()
            n285 = Array To Cluster(array=w988) -> (cluster=w990:T5)
            n286 = Unbundle(w990) -> ("[0]"=w989:cluster{dbl[], dbl[]})  [unwired: 8 out]
            n287 = local write "Threshold V"(w980) -> ()
            n288 = local write "S.T.S."(w974) -> ()
            n289 = Unbundle(w989) -> (w964:dbl[], w971:dbl[])
            n290 = local write "XY Graph"(w987) -> ()
            n291 = local write "Table Control 2"(w1017) -> ()
            n292 = local write "Mobility"(w1016) -> ()
            n293 = local write "Length"(w978) -> ()
            n294 = local write "XY Graph 2"(w965) -> ()
            n295 = Unbundle(w959) -> ("Vt"=w961:dbl, "STS"=w960:dbl, "On/Off"=w958:dbl)  [unwired: 4 out]
            n296 = local write "On/Off"(w958) -> ()
            n297 = Array Subset(array=w963, index=w970, length=w969) -> (w973:dbl[])
            n298 = Array Subset(array=w962, index=w970, length=w969) -> (w972:dbl[])
            n299 = local write "Width"(w952) -> ()
            n300 = Array Subset(array=w964, index=w984, length=w976) -> (w986:dbl[])
            n301 = Array Subset(array=w971, index=w984, length=w976) -> (w985:dbl[])
            n302 = local write "Array 8"(w973) -> ()
            n303 = local write "Array 7"(w972) -> ()
            n304 = local write "STS recorded"(w960) -> ()
            n305 = local write "Vt recorded"(w961) -> ()
            n306 = local write "New Length"(w978) -> ()
            n307 = local write "New Width"(w952) -> ()
            n308 = local write "Array 2"(w985) -> ()
            n309 = local write "Array"(w986) -> ()
            n310 = local write "Data File"(w977) -> ()
            n311 = local read "Image Folder"() -> (w943:path)
            n312 = local write "Index"(w984) -> ()
            n313 = local write "Slide"(w984) -> ()
            n314 = List Folder(path=w943, error in=w947) -> (filenames=w1001:string[], error out=w946:errorcluster)  [unwired: 2 in, 2 out]
            n315 = call-poly <vilib>:"Read From Spreadsheet File.vi"("file path (dialog if empty)"=w977) -> ("all rows"=w1010:string[][])  [unwired: 6 in, 4 out]
            n316 = Array Size(array=w1010) -> (size(s)=w1009:i32[])
            n317 = Index Array(array=w1009, index=w1008) -> (element=w983:i32)
            n318 = Subtract(x=w983, y=20) -> (x-y=w981:i32)
            n319 = property on="Slide" class="Slide (strict)"("Scale.Maximum"=w981) -> ()  [unwired: 2 in, 2 out]
            n320 = Array Subset(array=w1010, index (row)=w1008, index (col)=w1008, length (col)=3) -> (w1011:string[][])  [unwired: 1 in]
            n321 = Reshape Array(w1011, w983) -> (w991:string[])
            n322 = Search 1D Array(1D array=w991, element="Index:") -> (index of element=w1005:i32)  [unwired: 1 in]
            n323 = Increment(x=w1005) -> (x+1=w1006:i32)
            n324 = Index Array(array=w991, index=w1006) -> (element=w945:string)
            n325 = while {
              tunnel: w1001 -> [w1035]
              tunnel: w945 -> [w1033]
              tunnel: [w1032] -> _
              tunnel: [w1032] -> w1000
              tunnel: w983 -> [w1031]
              i -> [w1032]
              stop <- w1028 stop-if-true
              n326 = Index Array(array=w1035, index=w1032) -> (element=w1036:string)
              n327 = xnode "Match Regular Expression"("input string"=w1036, "regular expression"=w1033) -> ("whole match"=w1034:string)  [unwired: 4 in, 4 out]
              n328 = Equal?(x=w1034, y=w1033) -> (x = y?=w1030:bool)
              n329 = Equal?(x=w1031, y=w1032) -> (x = y?=w1029:bool)
              n330 = Or(x=w1030, y=w1029) -> (x .or. y?=w1028:bool)
            }
            n331 = local write "Index 3"(w945) -> ()
            n332 = Search 1D Array(1D array=w991, element="Mobility (cm^2/Vs):") -> (index of element=w996:i32)  [unwired: 1 in]
            n333 = Increment(x=w996) -> (x+1=w995:i32)
            n334 = Index Array(array=w991, index=w995) -> (element=w993:string)
            n335 = Fract/Exp String To Number(string=w993) -> (number=w992:dbl)  [unwired: 3 in, 1 out]
            n336 = local write "Recorded Mobility"(w992) -> ()
            n337 = Build Path(base path=w943, name or relative path="ROI") -> (appended path=w942:path)
            n338 = Path To String(path=w943) -> (string=w999:string)
            n339 = local read "No Image"() -> (w953:path)
            n340 = Build Path(base path=w942, name or relative path=w945) -> (appended path=w951:path)
            n341 = invoke on="Image Out" class="ImageControl" method="Clear ROI"(error in=w946) -> (error out=w950:errorcluster)  [unwired: 2 in, 2 out]
            n342 = Index Array(array=w1001, index=w1000) -> (element=w956:string)
            n343 = Empty String/Path?(string/path=w956) -> (empty?=w957:bool)
            n344 = Concatenate Strings(w999, "\\", w956) -> (w998:string)
            n345 = String To Path(string=w998) -> (path=w955:path)
            n346 = Select(t=w953, s=w957, f=w955) -> (s? t:f=w954:path)
            n347 = call "Vision Acquisition3"("Image Path"=w954) -> ("Image Out"=w1002:T2)  [unwired: 25 in, 1 out]
            n348 = local write "Image File"(w954) -> ()
            n349 = local write "Image Out 2"(w1002) -> ()
            n350 = local write "Image Out"(w1002) -> ()
            n351 = local write "Image Name"(w956) -> ()
            n352 = call <vilib>:"Check if File or Folder Exists.vi"("error in (no error)"=w950, "path"=w951) -> ("file or folder exists?"=w948:bool, "dup path"=w949:path)  [unwired: 7 in, 1 out]
            n353 = invoke on="Image Out" class="ImageControl" method="Clear ROI"() -> ()  [unwired: 3 in, 3 out]
            n354 = case shown="True" w948 {
              tunnel: w949 -> [_ w1023]
              frame False {
              }
              frame True {
                n355 = Read from Text File(file (use dialog)=w1023) -> (text=w1027:string)  [unwired: 3 in, 3 out]
                n356 = property on="Image Out" class="ImageControl"() -> ("ROI"=w1024:T7)  [unwired: 2 in, 2 out]
                n357 = Unflatten From String(type=w1024, binary string=w1027) -> (value=w1025:T7, error out=w1026:errorcluster)  [unwired: 3 in, 1 out]
                n358 = property on="Image Out" class="ImageControl"(error in=w1026, "ROI"=w1025) -> ()  [unwired: 1 in, 2 out]
              }
            }
          }
          event "Up Button": Mouse Down {
            w1219 = 0
            n359 = event-data() -> ()  [unwired: 1 in, 5 out]
            n360 = local read "NumPts"() -> (w1190:dbl)
            n361 = local read "Row Start"() -> (w1189:dbl)
            n362 = local read "Data File"() -> (w1215:path)
            n363 = local read "NumPts 2"() -> (w1184:dbl)
            n364 = property on="Image Out" class="ImageControl"() -> (error out=w1148:errorcluster, "Image Center Position"=w1152:cluster{"X":u32, "Y":u32})  [unwired: 2 in, 1 out]
            n365 = Strip Path(path=w1215) -> (stripped path=w1214:path, name=w1235:string)
            n366 = local write "Data Folder"(w1214) -> ()
            n367 = List Folder(path=w1214) -> (filenames=w1225:string[], error out=w1158:errorcluster)  [unwired: 3 in, 2 out]
            n368 = Path To String(path=w1214) -> (string=w1236:string)
            n369 = Search 1D Array(1D array=w1225, element=w1235) -> (index of element=w1227:i32)  [unwired: 1 in]
            n370 = Equal To 0?(x=w1227) -> (x = 0?=w1228:bool)
            n371 = Unbundle(w1152) -> ("X"=w1150:u32)  [unwired: 1 out]
            n372 = Bundle("X"=w1150, 0) -> (w1151:cluster{"X":u32, i32})  [unwired: 1 in]
            n373 = property on="Image Out" class="ImageControl"(error in=w1148, "Image Center Position"=w1151) -> ()  [unwired: 1 in, 2 out]
            n374 = Array Size(array=w1225) -> (size(s)=w1224:i32)
            n375 = case shown="True" w1228 {
              tunnel: w1227 -> [w1363 _]
              tunnel: [w1362 w1364] -> w1226
              tunnel: w1224 -> [_ w1365]
              frame False {
                n376 = Decrement(x=w1363) -> (x-1=w1362:i32)
              }
              frame True {
                n377 = Decrement(x=w1365) -> (x-1=w1364:i32)
              }
            }
            n378 = Index Array(array=w1225, index=w1226) -> (element=w1229:string)
            n379 = local write "Data Name"(w1229) -> ()
            n380 = Concatenate Strings(w1236, "\\", w1229) -> (w1234:string)
            n381 = String To Path(string=w1234) -> (path=w1191:path)
            n382 = call "sub_thresh_swing_subvi.vi"("Path"=w1191, "NumPts"=w1184, "Row Start"=w1189) -> ("Index"=w1183:dbl, "XY Graph"=w1179:cluster{dbl[], dbl[]}[], "Sub Threshold Swing"=w1192:dbl)  [unwired: 8 in, 2 out]
            n383 = Decimate 1D Array(w1179) -> (w1182:cluster{dbl[], dbl[]}[])  [unwired: 1 out]
            n384 = Array To Cluster(array=w1182) -> (cluster=w1180:T5)
            n385 = Unbundle(w1180) -> ("[0]"=w1181:cluster{dbl[], dbl[]})  [unwired: 8 out]
            n386 = Unbundle(w1181) -> (w1178:dbl[], w1177:dbl[])
            n387 = Array Subset(array=w1178, index=w1183, length=w1184) -> (w1186:dbl[])
            n388 = Array Subset(array=w1177, index=w1183, length=w1184) -> (w1185:dbl[])
            n389 = local write "S.T.S."(w1192) -> ()
            n390 = local write "Array 8"(w1186) -> ()
            n391 = local write "Array 7"(w1185) -> ()
            n392 = call "mobility_subvi.vi"("Path"=w1191, "NumPts"=w1190, "Row Start"=w1189) -> ("Dielectric (d)"=w1194:dbl, "Index"=w1196:dbl, "XY Graph"=w1202:cluster{dbl[], dbl[]}[], "Length"=w1193:dbl, "Vt"=w1195:dbl, "Width"=w1170:dbl, "Table Control"=w1232:string[][], "Table Control 2"=w1231:string[][], "Recorded"=w1174:T6, "Mobility"=w1230:dbl)  [unwired: 2 in, 1 out]
            n393 = local write "Dielectric (d)"(w1194) -> ()
            n394 = local write "New Dielectric"(w1194) -> ()
            n395 = local write "New Length"(w1193) -> ()
            n396 = local write "New Width"(w1170) -> ()
            n397 = local write "Table Control"(w1232) -> ()
            n398 = Decimate 1D Array(w1202) -> (w1203:cluster{dbl[], dbl[]}[])  [unwired: 1 out]
            n399 = local write "XY Graph 2"(w1179) -> ()
            n400 = Array To Cluster(array=w1203) -> (cluster=w1205:T5)
            n401 = local write "XY Graph"(w1202) -> ()
            n402 = local write "Index 2"(w1183) -> ()
            n403 = local write "Table Control 2"(w1231) -> ()
            n404 = local write "Mobility"(w1230) -> ()
            n405 = local write "Length"(w1193) -> ()
            n406 = Unbundle(w1205) -> ("[0]"=w1204:cluster{dbl[], dbl[]})  [unwired: 8 out]
            n407 = Unbundle(w1204) -> (w1188:dbl[], w1187:dbl[])
            n408 = local write "Threshold V"(w1195) -> ()
            n409 = local write "Width"(w1170) -> ()
            n410 = Unbundle(w1174) -> ("Vt"=w1176:dbl, "STS"=w1175:dbl, "On/Off"=w1173:dbl)  [unwired: 4 out]
            n411 = Array Subset(array=w1188, index=w1196, length=w1190) -> (w1201:dbl[])
            n412 = Array Subset(array=w1187, index=w1196, length=w1190) -> (w1200:dbl[])
            n413 = local write "STS recorded"(w1175) -> ()
            n414 = local write "Data File"(w1191) -> ()
            n415 = local write "Index"(w1196) -> ()
            n416 = local write "Vt recorded"(w1176) -> ()
            n417 = local write "On/Off"(w1173) -> ()
            n418 = local write "Array 2"(w1200) -> ()
            n419 = local write "Array"(w1201) -> ()
            n420 = local read "Image Folder"() -> (w1162:path)
            n421 = local write "Slide"(w1196) -> ()
            n422 = List Folder(path=w1162, error in=w1158) -> (filenames=w1213:string[], error out=w1157:errorcluster)  [unwired: 2 in, 2 out]
            n423 = call-poly <vilib>:"Read From Spreadsheet File.vi"("file path (dialog if empty)"=w1191) -> ("all rows"=w1221:string[][])  [unwired: 6 in, 4 out]
            n424 = Array Size(array=w1221) -> (size(s)=w1220:i32[])
            n425 = Index Array(array=w1220, index=w1219) -> (element=w1198:i32)
            n426 = Subtract(x=w1198, y=20) -> (x-y=w1197:i32)
            n427 = property on="Slide" class="Slide (strict)"("Scale.Maximum"=w1197) -> ()  [unwired: 2 in, 2 out]
            n428 = Array Subset(array=w1221, index (row)=w1219, index (col)=w1219, length (col)=3) -> (w1222:string[][])  [unwired: 1 in]
            n429 = Reshape Array(w1222, w1198) -> (w1208:string[])
            n430 = Search 1D Array(1D array=w1208, element="Mobility (cm^2/Vs):") -> (index of element=w1211:i32)  [unwired: 1 in]
            n431 = Increment(x=w1211) -> (x+1=w1210:i32)
            n432 = Index Array(array=w1208, index=w1210) -> (element=w1207:string)
            n433 = Fract/Exp String To Number(string=w1207) -> (number=w1206:dbl)  [unwired: 3 in, 1 out]
            n434 = local write "Recorded Mobility"(w1206) -> ()
            n435 = Search 1D Array(1D array=w1208, element="Index:") -> (index of element=w1216:i32)  [unwired: 1 in]
            n436 = Increment(x=w1216) -> (x+1=w1217:i32)
            n437 = Index Array(array=w1208, index=w1217) -> (element=w1154:string)
            n438 = while {
              tunnel: w1213 -> [w1249]
              tunnel: w1154 -> [w1247]
              tunnel: [w1246] -> w1212
              tunnel: w1198 -> [w1245]
              i -> [w1246]
              stop <- w1242 stop-if-true
              n439 = Index Array(array=w1249, index=w1246) -> (element=w1250:string)
              n440 = xnode "Match Regular Expression"("input string"=w1250, "regular expression"=w1247) -> ("whole match"=w1248:string)  [unwired: 4 in, 4 out]
              n441 = Equal?(x=w1248, y=w1247) -> (x = y?=w1244:bool)
              n442 = Equal?(x=w1245, y=w1246) -> (x = y?=w1243:bool)
              n443 = Or(x=w1244, y=w1243) -> (x .or. y?=w1242:bool)
            }
            n444 = local write "Index 3"(w1154) -> ()
            n445 = Build Path(base path=w1162, name or relative path="ROI") -> (appended path=w1155:path)
            n446 = Build Path(base path=w1155, name or relative path=w1154) -> (appended path=w1153:path)
            n447 = invoke on="Image Out" class="ImageControl" method="Clear ROI"(error in=w1157) -> (error out=w1161:errorcluster)  [unwired: 2 in, 2 out]
            n448 = call <vilib>:"Check if File or Folder Exists.vi"("error in (no error)"=w1161, "path"=w1153) -> ("file or folder exists?"=w1159:bool, "dup path"=w1160:path)  [unwired: 7 in, 1 out]
            n449 = local read "No Image"() -> (w1171:path)
            n450 = Index Array(array=w1213, index=w1212) -> (element=w1164:string)
            n451 = Build Path(base path=w1162, name or relative path=w1164) -> (appended path=w1163:path)
            n452 = local write "Image Name"(w1164) -> ()
            n453 = Empty String/Path?(string/path=w1164) -> (empty?=w1172:bool)
            n454 = case shown="True" w1159 {
              tunnel: w1160 -> [_ w1237]
              frame False {
              }
              frame True {
                n455 = Read from Text File(file (use dialog)=w1237) -> (text=w1241:string)  [unwired: 3 in, 3 out]
                n456 = property on="Image Out" class="ImageControl"() -> ("ROI"=w1238:T7)  [unwired: 2 in, 2 out]
                n457 = Unflatten From String(type=w1238, binary string=w1241) -> (value=w1239:T7, error out=w1240:errorcluster)  [unwired: 3 in, 1 out]
                n458 = property on="Image Out" class="ImageControl"(error in=w1240, "ROI"=w1239) -> ()  [unwired: 1 in, 2 out]
              }
            }
            n459 = Select(t=w1171, s=w1172, f=w1163) -> (s? t:f=w1165:path)
            n460 = call "Vision Acquisition5"("Image Path"=w1165) -> ("Image Out"=w1169:T2)  [unwired: 25 in, 1 out]
            n461 = local write "Image File"(w1165) -> ()
            n462 = local write "Image Out 2"(w1169) -> ()
            n463 = local write "Image Out"(w1169) -> ()
            n464 = call <vilib>:"Get File Extension.vi"("file"=w1165) -> ("lowercase file extension"=w1167:string)  [unwired: 7 in, 3 out]
            n465 = local write "String"(w1167) -> ()
            n466 = Search 1D Array(1D array=string[] ["bmp", "jpeg", "png", "jpg", "gif"], element=w1167) -> (index of element=w1166:i32)  [unwired: 1 in]
            n467 = Less Than 0?(x=w1166) -> ()  [unwired: 1 out]
          }
          event "Save Changes? 3": Mouse Down {
            n468 = event-data() -> ()  [unwired: 1 in, 7 out]
            n469 = local read "Image Folder"() -> (w1366:path)
            n470 = Build Path(base path=w1366, name or relative path="ROI") -> (appended path=w1373:path)
            n471 = call <vilib>:"Check if File or Folder Exists.vi"("path"=w1373) -> ("file or folder exists?"=w1375:bool, "dup path"=w1372:path)  [unwired: 8 in, 1 out]
            n472 = case shown="False" w1375 {
              tunnel: w1372 -> [w1377 w1378]
              tunnel: [w1376 w1378] -> w1367
              frame False {
                n473 = Create Folder(path (use dialog)=w1377) -> (created path=w1376:path)  [unwired: 2 in, 2 out]
              }
              frame True {
              }
            }
            n474 = property on="Image Out" class="ImageControl"() -> ("ROI"=w1371:T7)  [unwired: 2 in, 2 out]
            n475 = local read "Index 3"() -> (w1369:string)
            n476 = Flatten To String(anything=w1371) -> (data string=w1370:string)  [unwired: 3 in, 2 out]
            n477 = Build Path(base path=w1367, name or relative path=w1369) -> (appended path=w1368:path)
            n478 = Write to Text File(file (use dialog)=w1368, text=w1370) -> ()  [unwired: 2 in, 3 out]
          }
          event "Next Button": Mouse Down {
            n479 = event-data() -> ()  [unwired: 1 in, 5 out]
            n480 = local read "XY Graph"() -> (w1391:cluster{dbl[], dbl[]}[])
            n481 = local read "NumPts"() -> (w1392:dbl)
            n482 = local read "Index"() -> (w1393:dbl)
            n483 = Decimate 1D Array(w1391) -> (w1387:cluster{dbl[], dbl[]}[], w1386:cluster{dbl[], dbl[]}[])
            n484 = Array To Cluster(array=w1387) -> (cluster=w1397:T5)
            n485 = Unbundle(w1397) -> ("[0]"=w1396:cluster{dbl[], dbl[]})  [unwired: 8 out]
            n486 = Increment(x=w1393) -> (x+1=w1388:dbl)
            n487 = Unbundle(w1396) -> (w1395:dbl[], w1394:dbl[])
            n488 = Array Subset(array=w1395, index=w1388, length=w1392) -> (w1384:dbl[])
            n489 = local write "Index"(w1388) -> ()
            n490 = Array Subset(array=w1394, index=w1388, length=w1392) -> (w1383:dbl[])
            n491 = Bundle(w1384, w1383) -> (w1390:cluster{dbl[], dbl[]})  [unwired: 1 in]
            n492 = Build Array (concatenate)(w1387, w1386, w1390) -> (w1389:cluster{dbl[], dbl[]}[])
            n493 = local write "XY Graph"(w1389) -> ()
            n494 = local read "New Dielectric"() -> (w1382:dbl)
            n495 = local write "Array 2"(w1383) -> ()
            n496 = local read "New Length"() -> (w1381:dbl)
            n497 = local write "Array"(w1384) -> ()
            n498 = local read "New Width"() -> (w1380:dbl)
            n499 = call "mob_calc_subvi.vi"("Width"=w1380, "Length"=w1381, "Dielectric (d)"=w1382, "Array 2"=w1383, "Array"=w1384) -> ("Vt"=w1379:dbl, "Mobility"=w1385:dbl)  [unwired: 5 in]
            n500 = local write "New Mobility"(w1385) -> ()
            n501 = local write "New Vt"(w1379) -> ()
          }
          event "Next Button 2": Mouse Down {
            n502 = event-data() -> ()  [unwired: 1 in, 7 out]
            n503 = local read "XY Graph 2"() -> (w1406:cluster{dbl[], dbl[]}[])
            n504 = local read "Index 2"() -> (w1408:dbl)
            n505 = local read "NumPts 2"() -> (w1407:dbl)
            n506 = Decimate 1D Array(w1406) -> (w1402:cluster{dbl[], dbl[]}[], w1401:cluster{dbl[], dbl[]}[])
            n507 = Array To Cluster(array=w1402) -> (cluster=w1412:T5)
            n508 = Unbundle(w1412) -> ("[0]"=w1411:cluster{dbl[], dbl[]})  [unwired: 8 out]
            n509 = Increment(x=w1408) -> (x+1=w1403:dbl)
            n510 = Unbundle(w1411) -> (w1410:dbl[], w1409:dbl[])
            n511 = local write "Index 2"(w1403) -> ()
            n512 = Array Subset(array=w1410, index=w1403, length=w1407) -> (w1399:dbl[])
            n513 = Array Subset(array=w1409, index=w1403, length=w1407) -> (w1398:dbl[])
            n514 = Bundle(w1399, w1398) -> (w1405:cluster{dbl[], dbl[]})  [unwired: 1 in]
            n515 = Build Array (concatenate)(w1402, w1401, w1405) -> (w1404:cluster{dbl[], dbl[]}[])
            n516 = local write "XY Graph 2"(w1404) -> ()
            n517 = local write "Array 8"(w1399) -> ()
            n518 = call "sts_calc_subvi.vi"("Array 2"=w1399, "Array"=w1398) -> ("STS"=w1400:dbl)  [unwired: 9 in]
            n519 = local write "Array 7"(w1398) -> ()
            n520 = local write "New S.T.S."(w1400) -> ()
          }
          event "Previous Button 2": Mouse Down {
            n521 = event-data() -> ()  [unwired: 1 in, 7 out]
            n522 = local read "XY Graph 2"() -> (w1422:cluster{dbl[], dbl[]}[])
            n523 = local read "NumPts 2"() -> (w1423:dbl)
            n524 = local read "Index 2"() -> (w1415:dbl)
            n525 = Decimate 1D Array(w1422) -> (w1419:cluster{dbl[], dbl[]}[], w1418:cluster{dbl[], dbl[]}[])
            n526 = Array To Cluster(array=w1419) -> (cluster=w1427:T5)
            n527 = Unbundle(w1427) -> ("[0]"=w1426:cluster{dbl[], dbl[]})  [unwired: 8 out]
            n528 = Decrement(x=w1415) -> (x-1=w1416:dbl)
            n529 = Unbundle(w1426) -> (w1425:dbl[], w1424:dbl[])
            n530 = local write "Index 2"(w1416) -> ()
            n531 = Array Subset(array=w1425, index=w1416, length=w1423) -> (w1413:dbl[])
            n532 = Array Subset(array=w1424, index=w1416, length=w1423) -> (w1414:dbl[])
            n533 = Bundle(w1413, w1414) -> (w1421:cluster{dbl[], dbl[]})  [unwired: 1 in]
            n534 = Build Array (concatenate)(w1419, w1418, w1421) -> (w1420:cluster{dbl[], dbl[]}[])
            n535 = local write "XY Graph 2"(w1420) -> ()
            n536 = local write "Array 7"(w1414) -> ()
            n537 = call "sts_calc_subvi.vi"("Array 2"=w1413, "Array"=w1414) -> ("STS"=w1417:dbl)  [unwired: 9 in]
            n538 = local write "Array 8"(w1413) -> ()
            n539 = local write "New S.T.S."(w1417) -> ()
          }
          event "Previous Button": Mouse Down {
            n540 = event-data() -> ()  [unwired: 1 in, 5 out]
            n541 = local read "XY Graph"() -> (w1441:cluster{dbl[], dbl[]}[])
            n542 = Decimate 1D Array(w1441) -> (w1438:cluster{dbl[], dbl[]}[], w1437:cluster{dbl[], dbl[]}[])
            n543 = local read "NumPts"() -> (w1442:dbl)
            n544 = local read "Index"() -> (w1436:dbl)
            n545 = Array To Cluster(array=w1438) -> (cluster=w1446:T5)
            n546 = Unbundle(w1446) -> ("[0]"=w1445:cluster{dbl[], dbl[]})  [unwired: 8 out]
            n547 = Decrement(x=w1436) -> (x-1=w1435:dbl)
            n548 = Unbundle(w1445) -> (w1444:dbl[], w1443:dbl[])
            n549 = local read "New Dielectric"() -> (w1429:dbl)
            n550 = Array Subset(array=w1444, index=w1435, length=w1442) -> (w1434:dbl[])
            n551 = Array Subset(array=w1443, index=w1435, length=w1442) -> (w1433:dbl[])
            n552 = local write "Index"(w1435) -> ()
            n553 = Bundle(w1434, w1433) -> (w1440:cluster{dbl[], dbl[]})  [unwired: 1 in]
            n554 = Build Array (concatenate)(w1438, w1437, w1440) -> (w1439:cluster{dbl[], dbl[]}[])
            n555 = local write "XY Graph"(w1439) -> ()
            n556 = local read "New Length"() -> (w1430:dbl)
            n557 = local write "Array 2"(w1433) -> ()
            n558 = local read "New Width"() -> (w1431:dbl)
            n559 = call "mob_calc_subvi.vi"("Width"=w1431, "Length"=w1430, "Dielectric (d)"=w1429, "Array 2"=w1433, "Array"=w1434) -> ("Vt"=w1428:dbl, "Mobility"=w1432:dbl)  [unwired: 5 in]
            n560 = local write "New Mobility"(w1432) -> ()
            n561 = local write "Array"(w1434) -> ()
            n562 = local write "New Vt"(w1428) -> ()
          }
          event "Slide": Value Change {
            n563 = event-data() -> ()  [unwired: 1 in, 5 out]
            n564 = local read "XY Graph"() -> (w1459:cluster{dbl[], dbl[]}[])
            n565 = local read "Slide"() -> (w1448:dbl)
            n566 = Decimate 1D Array(w1459) -> (w1456:cluster{dbl[], dbl[]}[], w1455:cluster{dbl[], dbl[]}[])
            n567 = local read "NumPts"() -> (w1460:dbl)
            n568 = Array To Cluster(array=w1456) -> (cluster=w1464:T5)
            n569 = Unbundle(w1464) -> ("[0]"=w1463:cluster{dbl[], dbl[]})  [unwired: 8 out]
            n570 = Unbundle(w1463) -> (w1462:dbl[], w1461:dbl[])
            n571 = local read "New Dielectric"() -> (w1449:dbl)
            n572 = Array Subset(array=w1462, index=w1448, length=w1460) -> (w1454:dbl[])
            n573 = Array Subset(array=w1461, index=w1448, length=w1460) -> (w1453:dbl[])
            n574 = local write "Index"(w1448) -> ()
            n575 = Bundle(w1454, w1453) -> (w1458:cluster{dbl[], dbl[]})  [unwired: 1 in]
            n576 = Build Array (concatenate)(w1456, w1455, w1458) -> (w1457:cluster{dbl[], dbl[]}[])
            n577 = local write "XY Graph"(w1457) -> ()
            n578 = local read "New Length"() -> (w1450:dbl)
            n579 = local write "Array 2"(w1453) -> ()
            n580 = local read "New Width"() -> (w1451:dbl)
            n581 = call "mob_calc_subvi.vi"("Width"=w1451, "Length"=w1450, "Dielectric (d)"=w1449, "Array 2"=w1453, "Array"=w1454) -> ("Vt"=w1447:dbl, "Mobility"=w1452:dbl)  [unwired: 5 in]
            n582 = local write "New Mobility"(w1452) -> ()
            n583 = local write "Array"(w1454) -> ()
            n584 = local write "New Vt"(w1447) -> ()
          }
          event "Slide 2": Value Change {
            n585 = event-data() -> ()  [unwired: 1 in, 5 out]
            n586 = local read "XY Graph 2"() -> (w1473:cluster{dbl[], dbl[]}[])
            n587 = local read "Slide 2"() -> (w1468:dbl)
            n588 = Decimate 1D Array(w1473) -> (w1470:cluster{dbl[], dbl[]}[], w1469:cluster{dbl[], dbl[]}[])
            n589 = local read "NumPts 2"() -> (w1474:dbl)
            n590 = Array To Cluster(array=w1470) -> (cluster=w1478:T5)
            n591 = Unbundle(w1478) -> ("[0]"=w1477:cluster{dbl[], dbl[]})  [unwired: 8 out]
            n592 = Unbundle(w1477) -> (w1476:dbl[], w1475:dbl[])
            n593 = Array Subset(array=w1476, index=w1468, length=w1474) -> (w1466:dbl[])
            n594 = Array Subset(array=w1475, index=w1468, length=w1474) -> (w1465:dbl[])
            n595 = local write "Index 2"(w1468) -> ()
            n596 = Bundle(w1466, w1465) -> (w1472:cluster{dbl[], dbl[]})  [unwired: 1 in]
            n597 = Build Array (concatenate)(w1470, w1469, w1472) -> (w1471:cluster{dbl[], dbl[]}[])
            n598 = local write "XY Graph 2"(w1471) -> ()
            n599 = local write "Array 7"(w1465) -> ()
            n600 = local write "Array 8"(w1466) -> ()
            n601 = call "sts_calc_subvi.vi"("Array 2"=w1466, "Array"=w1465) -> ("STS"=w1467:dbl)  [unwired: 9 in]
            n602 = local write "New S.T.S."(w1467) -> ()
          }
          event "Save Changes?": Mouse Down {
            n603 = event-data() -> ()  [unwired: 1 in, 5 out]
            n604 = Build Array("DeviceID", "Fabricator", "Deposition", "Date", "Sample", "Row", "Column", "L", "W", "Material", "Treatment", "Treatment Concentration", "Solvent", "Concentration", "ST (C)", "Drops", "RT (F)", "RH (%)", "RPM", "Accel (RPM/s)", "Time", "Mobility", "On/Off", "Vt", "S.T.S") -> (w1480:string[])
            "Export \nHeaders" <- w1480
            n605 = flat-sequence {
              tunnel: [w1595] -> w1512
              tunnel: [w1594] -> w1510
              tunnel: [w1594] -> w1509
              tunnel: [w1577] -> w1507
              tunnel: [w1513] -> w1479
              tunnel: w1512 -> [w1656]
              tunnel: [w1657] -> w1511
              tunnel: w1510 -> [w1657]
              tunnel: w1509 -> [w1655]
              tunnel: [w1653] -> w1508
              tunnel: w1507 -> [w1653]
              tunnel: w1511 -> [w1662]
              tunnel: w1508 -> [w1661]
              frame #0 {
                w1547 = "/"
                w1582 = -1
                w1575 = "S.T.S. (V/decade):"
                w1576 = "Threshold V (V):"
                (unwired) 3
                w1580 = 1
                n606 = local read "Data File"() -> (w1595:path)
                n607 = local read "New Dielectric"() -> (w1618:dbl)
                n608 = local read "New Width"() -> (w1608:dbl)
                n609 = local read "New Length"() -> (w1606:dbl)
                n610 = local read "New Mobility"() -> (w1617:dbl)
                n611 = local read "Index 3"() -> (w1527:string)
                n612 = local read "Date Recorded"() -> (w1550:string)
                n613 = String Subset(string=w1527, length (rest)=1) -> (substring=w1524:string)  [unwired: 1 in]
                n614 = local write "Row"(w1524) -> ()
                n615 = Match Pattern(string=w1550, regular expression=w1547) -> (before substring=w1541:string, after substring=w1548:string)  [unwired: 1 in, 2 out]
                n616 = call-poly <vilib>:"Read From Spreadsheet File.vi"("file path (dialog if empty)"=w1595) -> ("all rows"=w1587:string[][])  [unwired: 6 in, 4 out]
                n617 = String Length(string=w1541) -> (length=w1544:i32)
                n618 = Match Pattern(string=w1548, regular expression=w1547) -> (before substring=w1535:string, after substring=w1546:string)  [unwired: 1 in, 2 out]
                n619 = String Subset(string=w1527, offset (0)=1, length (rest)=2) -> (substring=w1525:string)
                n620 = Number To Fractional String(number=w1606) -> (F-format string=w1598:string)  [unwired: 3 in]
                n621 = Replace Array Subset(array=w1587, new element=w1598, index (row)=12, index (col)=w1580) -> (w1602:string[][])
                n622 = Number To Fractional String(number=w1608) -> (F-format string=w1609:string)  [unwired: 3 in]
                n623 = Replace Array Subset(array=w1602, new element=w1609, index (row)=13, index (col)=w1580) -> (w1604:string[][])
                n624 = Number To Fractional String(number=w1617) -> (F-format string=w1596:string)  [unwired: 3 in]
                n625 = Number To Fractional String(number=w1618) -> (F-format string=w1597:string)  [unwired: 3 in]
                n626 = Number To Decimal String(number=w1606) -> (decimal integer string=w1605:string)  [unwired: 1 in]
                n627 = String Length(string=w1535) -> (length=w1537:i32)
                n628 = local read "Index 3"() -> (w1534:string)
                n629 = Equal?(x=w1544, y=2) -> (x = y?=w1542:bool)
                n630 = case shown="False" w1542 {
                  tunnel: w1541 -> [w1624 w1626]
                  tunnel: [w1623 w1626] -> w1540
                  frame False {
                    n631 = Concatenate Strings("0", w1624) -> (w1623:string)
                  }
                  frame True {
                  }
                }
                n632 = local write "Column"(w1525) -> ()
                n633 = Strip Path(path=w1595) -> (stripped path=w1616:path)  [unwired: 1 out]
                n634 = local read "Index 3"() -> (w1611:string)
                n635 = Replace Array Subset(array=w1604, new element=w1596, index (row)=15, index (col)=w1580) -> (w1603:string[][])
                n636 = Number To Decimal String(number=w1608) -> (decimal integer string=w1607:string)  [unwired: 1 in]
                n637 = Equal?(x=w1537, y=2) -> (x = y?=w1539:bool)
                n638 = local read "Relative Humidity (%):"() -> (w1516:dbl)
                n639 = Path To String(path=w1616) -> (string=w1614:string)
                n640 = case shown="False" w1539 {
                  tunnel: w1535 -> [w1620 w1622]
                  tunnel: [w1619 w1622] -> w1536
                  frame False {
                    n641 = Concatenate Strings("0", w1620) -> (w1619:string)
                  }
                  frame True {
                  }
                }
                n642 = Replace Array Subset(array=w1603, new element=w1597, index (row)=7, index (col)=w1580) -> (w1579:string[][])
                n643 = call "Build Text"("Index"=w1611, "Length"=w1605, "Width"=w1607) -> ("Result"=w1612:string)  [unwired: 11 in, 1 out]
                n644 = Concatenate Strings(w1614, "\\", w1612) -> (w1613:string)
                n645 = String To Path(string=w1613) -> (path=w1594:path)
                n646 = local read "Treatment Concentration (mM):"() -> (w1519:dbl)
                n647 = Number To Decimal String(number=w1516) -> (decimal integer string=w1515:string)  [unwired: 1 in]
                n648 = local read "Solution Temp (C):"() -> (w1569:dbl)
                n649 = local read "Surface Treatment:"() -> (w1518:string)
                n650 = local read "Material Recorded"() -> (w1514:string)
                n651 = local read "Room Temp (F):"() -> (w1573:dbl)
                n652 = local read "Concentration Recorded"() -> (w1521:string)
                n653 = local read "Accel (RPM/s):"() -> (w1560:dbl)
                n654 = local read "New Mobility"() -> (w1562:dbl)
                n655 = local read "New Length"() -> (w1533:dbl)
                n656 = local read "New Width"() -> (w1532:dbl)
                n657 = local read "Sample #:"() -> (w1552:dbl)
                n658 = local read "New S.T.S."() -> (w1554:dbl)
                n659 = local read "Method Recorded"() -> (w1553:string)
                n660 = local read "Time (s):"() -> (w1565:dbl)
                n661 = local read "# Drops:"() -> (w1570:dbl)
                n662 = local read "Solvent Recorded"() -> (w1520:string)
                n663 = local read "On/Off"() -> (w1558:dbl)
                n664 = local read "New Vt"() -> (w1556:dbl)
                n665 = local read "Date Recorded"() -> (w1549:string)
                n666 = local read "RPM:"() -> (w1566:dbl)
                n667 = local read "Fabricator:"() -> (w1574:string)
                n668 = local read "Column"() -> (w1523:string)
                n669 = Number To Decimal String(number=w1552) -> (decimal integer string=w1545:string)  [unwired: 1 in]
                n670 = call "DeviceID"("Sample"=w1545, "Year"=w1546, "Month"=w1540, "Day"=w1536, "Index"=w1534) -> ("Result"=w1551:string)  [unwired: 9 in, 1 out]
                n671 = Number To Decimal String(number=w1533) -> (decimal integer string=w1531:string)  [unwired: 1 in]
                n672 = Number To Decimal String(number=w1532) -> (decimal integer string=w1530:string)  [unwired: 1 in]
                n673 = Number To Decimal String(number=w1569) -> (decimal integer string=w1568:string)  [unwired: 1 in]
                n674 = Number To Decimal String(number=w1570) -> (decimal integer string=w1571:string)  [unwired: 1 in]
                n675 = Number To Decimal String(number=w1573) -> (decimal integer string=w1572:string)  [unwired: 1 in]
                n676 = Number To Decimal String(number=w1566) -> (decimal integer string=w1567:string)  [unwired: 1 in]
                n677 = Number To Fractional String(number=w1560) -> (F-format string=w1561:string)  [unwired: 3 in]
                n678 = Number To Decimal String(number=w1565) -> (decimal integer string=w1564:string)  [unwired: 1 in]
                n679 = Number To Fractional String(number=w1562) -> (F-format string=w1563:string)  [unwired: 3 in]
                n680 = Number To Fractional String(number=w1558) -> (F-format string=w1559:string)  [unwired: 3 in]
                n681 = Number To Fractional String(number=w1556) -> (F-format string=w1557:string)  [unwired: 3 in]
                n682 = Number To Fractional String(number=w1554) -> (F-format string=w1555:string)  [unwired: 3 in]
                n683 = Number To Decimal String(number=w1519) -> (decimal integer string=w1517:string)  [unwired: 1 in]
                n684 = Array Size(array=w1587) -> (size(s)=w1589:i32[])
                n685 = Index Array(array=w1589, index=0) -> (element=w1588:i32)
                n686 = local read "Row"() -> (w1522:string)
                n687 = Array Subset(array=w1587, index (row)=0, index (col)=0) -> (w1593:string[][])  [unwired: 2 in]
                n688 = Build Array(w1551, w1574, w1553, w1549, w1545, w1522, w1523, w1531, w1530, w1514, w1518, w1517, w1520, w1521, w1568, w1571, w1572, w1515, w1567, w1561, w1564, w1563, w1559, w1557, w1555) -> (w1513:string[])
                "Current\nRecord" <- w1513
                n689 = Reshape Array(w1593, w1588) -> (w1581:string[])
                n690 = Search 1D Array(1D array=w1581, element=w1576) -> (index of element=w1585:i32)  [unwired: 1 in]
                n691 = Search 1D Array(1D array=w1581, element=w1575) -> (index of element=w1586:i32)  [unwired: 1 in]
                n692 = Equal?(x=w1585, y=w1582) -> (x = y?=w1583:bool)
                n693 = Equal?(x=w1586, y=w1582) -> (x = y?=w1584:bool)
                n694 = case shown="True" w1583 {
                  tunnel: w1585 -> [_ _]
                  tunnel: w1579 -> [w1643 w1651]
                  tunnel: [w1642 w1650] -> w1578
                  tunnel: w1576 -> [_ w1649]
                  frame False {
                    n695 = local read "New Vt"() -> (w1645:dbl)
                    n696 = Number To Fractional String(number=w1645) -> (F-format string=w1641:string)  [unwired: 3 in]
                    n697 = Replace Array Subset(array=w1643, new element=w1641, index (row)=17, index (col)=1) -> (w1642:string[][])
                  }
                  frame True {
                    n698 = local read "New Vt"() -> (w1652:dbl)
                    n699 = Number To Fractional String(number=w1652) -> (F-format string=w1648:string)  [unwired: 3 in]
                    n700 = Build Array(w1649, w1648) -> (w1647:string[])
                    n701 = Insert Into Array(array=w1651, index (row)=17, new element=w1647) -> (w1650:string[][])  [unwired: 1 in]
                  }
                }
                n702 = case shown="True" w1584 {
                  tunnel: w1586 -> [_ _]
                  tunnel: w1578 -> [w1630 w1638]
                  tunnel: [w1629 w1637] -> w1577
                  tunnel: w1575 -> [_ w1635]
                  frame False {
                    n703 = local read "New S.T.S."() -> (w1632:dbl)
                    n704 = Number To Fractional String(number=w1632) -> (F-format string=w1628:string)  [unwired: 3 in]
                    n705 = Replace Array Subset(array=w1630, new element=w1628, index (row)=18, index (col)=1) -> (w1629:string[][])
                  }
                  frame True {
                    n706 = local read "New S.T.S."() -> (w1639:dbl)
                    n707 = Number To Fractional String(number=w1639) -> (F-format string=w1636:string)  [unwired: 3 in]
                    n708 = Build Array(w1635, w1636) -> (w1634:string[])
                    n709 = Insert Into Array(array=w1638, index (row)=18, new element=w1634) -> (w1637:string[][])  [unwired: 1 in]
                  }
                }
              }
              frame #1 {
                n710 = Equal?(x=w1656, y=w1655) -> (x = y?=w1654:bool)
                n711 = case shown="False" w1654 {
                  tunnel: w1656 -> [w1660 _]
                  tunnel: w1655 -> [w1659 _]
                  frame False {
                    n712 = Move(source path=w1660, 9:TRUE, 10:w1659) -> ()  [unwired: 2 in, 3 out]
                  }
                  frame True {
                  }
                }
              }
              frame #2 {
                n713 = local write "Data File"(w1662) -> ()
                n714 = call-poly <vilib>:"Write To Spreadsheet File.vi"("2D data"=w1661, "file path (dialog if empty)"=w1662) -> ()  [unwired: 6 in, 1 out]
              }
            }
            n715 = Build Array(w1480, w1479) -> (→"Full Database":string[][])
          }
          event "Save Changes? 2": Mouse Down {
            n716 = event-data() -> ()  [unwired: 1 in, 5 out]
            n717 = stacked-sequence {
              seq-local: [w1683 _ _ _ _] -> [_ w1736 _ _ _]
              seq-local: [w1682 _ _ _ _] -> [_ w1737 _ _ _]
              seq-local: [w1682 _ _ _ _] -> [_ w1735 _ _ _]
              seq-local: [w1665 _ _ _ _] -> [_ w1733 _ _ _]
              seq-local: [_ w1737 _ _ _] -> [_ _ w1742 _ _]
              seq-local: [_ w1733 _ _ _] -> [_ _ w1741 _ _]
              frame #0 {
                w1670 = -1
                w1663 = "S.T.S. (V/decade):"
                w1664 = "Threshold V (V):"
                (unwired) 3
                w1668 = 1
                n718 = local read "Data File"() -> (w1683:path)
                n719 = local read "New Width"() -> (w1696:dbl)
                n720 = local read "New Dielectric"() -> (w1706:dbl)
                n721 = local read "New Length"() -> (w1694:dbl)
                n722 = local read "New Mobility"() -> (w1705:dbl)
                n723 = call-poly <vilib>:"Read From Spreadsheet File.vi"("file path (dialog if empty)"=w1683) -> ("all rows"=w1675:string[][])  [unwired: 6 in, 4 out]
                n724 = Number To Fractional String(number=w1694) -> (F-format string=w1686:string)  [unwired: 3 in]
                n725 = Replace Array Subset(array=w1675, new element=w1686, index (row)=12, index (col)=w1668) -> (w1690:string[][])
                n726 = Number To Fractional String(number=w1696) -> (F-format string=w1697:string)  [unwired: 3 in]
                n727 = Replace Array Subset(array=w1690, new element=w1697, index (row)=13, index (col)=w1668) -> (w1692:string[][])
                n728 = Number To Fractional String(number=w1705) -> (F-format string=w1684:string)  [unwired: 3 in]
                n729 = Number To Fractional String(number=w1706) -> (F-format string=w1685:string)  [unwired: 3 in]
                n730 = Number To Decimal String(number=w1694) -> (decimal integer string=w1693:string)  [unwired: 1 in]
                n731 = Strip Path(path=w1683) -> (stripped path=w1704:path)  [unwired: 1 out]
                n732 = local read "Index 3"() -> (w1699:string)
                n733 = Replace Array Subset(array=w1692, new element=w1684, index (row)=15, index (col)=w1668) -> (w1691:string[][])
                n734 = Number To Decimal String(number=w1696) -> (decimal integer string=w1695:string)  [unwired: 1 in]
                n735 = Path To String(path=w1704) -> (string=w1702:string)
                n736 = Replace Array Subset(array=w1691, new element=w1685, index (row)=7, index (col)=w1668) -> (w1667:string[][])
                n737 = call "Build Text2"("Index"=w1699, "Length"=w1693, "Width"=w1695) -> ("Result"=w1700:string)  [unwired: 11 in, 1 out]
                n738 = Concatenate Strings(w1702, "\\", w1700) -> (w1701:string)
                n739 = String To Path(string=w1701) -> (path=w1682:path)
                n740 = Array Size(array=w1675) -> (size(s)=w1677:i32[])
                n741 = Index Array(array=w1677, index=0) -> (element=w1676:i32)
                n742 = Array Subset(array=w1675, index (row)=0, index (col)=0) -> (w1681:string[][])  [unwired: 2 in]
                n743 = Reshape Array(w1681, w1676) -> (w1669:string[])
                n744 = Search 1D Array(1D array=w1669, element=w1664) -> (index of element=w1673:i32)  [unwired: 1 in]
                n745 = Search 1D Array(1D array=w1669, element=w1663) -> (index of element=w1674:i32)  [unwired: 1 in]
                n746 = Equal?(x=w1673, y=w1670) -> (x = y?=w1671:bool)
                n747 = Equal?(x=w1674, y=w1670) -> (x = y?=w1672:bool)
                n748 = case shown="True" w1671 {
                  tunnel: w1673 -> [_ _]
                  tunnel: w1667 -> [w1723 w1731]
                  tunnel: [w1722 w1730] -> w1666
                  tunnel: w1664 -> [_ w1729]
                  frame False {
                    n749 = local read "New Vt"() -> (w1725:dbl)
                    n750 = Number To Fractional String(number=w1725) -> (F-format string=w1721:string)  [unwired: 3 in]
                    n751 = Replace Array Subset(array=w1723, new element=w1721, index (row)=17, index (col)=1) -> (w1722:string[][])
                  }
                  frame True {
                    n752 = local read "New Vt"() -> (w1732:dbl)
                    n753 = Number To Fractional String(number=w1732) -> (F-format string=w1728:string)  [unwired: 3 in]
                    n754 = Build Array(w1729, w1728) -> (w1727:string[])
                    n755 = Insert Into Array(array=w1731, index (row)=17, new element=w1727) -> (w1730:string[][])  [unwired: 1 in]
                  }
                }
                n756 = case shown="True" w1672 {
                  tunnel: w1674 -> [_ _]
                  tunnel: w1666 -> [w1710 w1718]
                  tunnel: [w1709 w1717] -> w1665
                  tunnel: w1663 -> [_ w1715]
                  frame False {
                    n757 = local read "New S.T.S."() -> (w1712:dbl)
                    n758 = Number To Fractional String(number=w1712) -> (F-format string=w1708:string)  [unwired: 3 in]
                    n759 = Replace Array Subset(array=w1710, new element=w1708, index (row)=18, index (col)=1) -> (w1709:string[][])
                  }
                  frame True {
                    n760 = local read "New S.T.S."() -> (w1719:dbl)
                    n761 = Number To Fractional String(number=w1719) -> (F-format string=w1716:string)  [unwired: 3 in]
                    n762 = Build Array(w1715, w1716) -> (w1714:string[])
                    n763 = Insert Into Array(array=w1718, index (row)=18, new element=w1714) -> (w1717:string[][])  [unwired: 1 in]
                  }
                }
              }
              frame #1 {
                n764 = Equal?(x=w1736, y=w1735) -> (x = y?=w1734:bool)
                n765 = case shown="False" w1734 {
                  tunnel: w1736 -> [w1740 _]
                  tunnel: w1735 -> [w1739 _]
                  frame False {
                    n766 = Move(source path=w1740, 9:TRUE, 10:w1739) -> ()  [unwired: 2 in, 3 out]
                  }
                  frame True {
                  }
                }
              }
              frame #2 {
                n767 = local write "Data File"(w1742) -> ()
                n768 = call-poly <vilib>:"Write To Spreadsheet File.vi"("2D data"=w1741, "file path (dialog if empty)"=w1742) -> ()  [unwired: 6 in, 1 out]
              }
              frame #3 {
                w1806 = 0
                n769 = local read "NumPts 2"() -> (w1765:dbl)
                n770 = local read "NumPts"() -> (w1772:dbl)
                n771 = local read "Row Start"() -> (w1771:dbl)
                n772 = local read "Data File"() -> (w1811:path)
                n773 = property on="Image Out" class="ImageControl"() -> (error out=w1746:errorcluster, "Image Center Position"=w1750:cluster{"X":u32, "Y":u32})  [unwired: 2 in, 1 out]
                n774 = Strip Path(path=w1811) -> (stripped path=w1802:path, name=w1824:string)
                n775 = local write "Data Folder"(w1802) -> ()
                n776 = List Folder(path=w1802) -> (filenames=w1817:string[])  [unwired: 3 in, 3 out]
                n777 = Unbundle(w1750) -> ("X"=w1748:u32)  [unwired: 1 out]
                n778 = Array Size(array=w1817) -> (size(s)=w1812:i32)
                n779 = Path To String(path=w1802) -> (string=w1825:string)
                n780 = Search 1D Array(1D array=w1817, element=w1824) -> (index of element=w1814:i32)  [unwired: 1 in]
                n781 = Bundle("X"=w1748, 0) -> (w1749:cluster{"X":u32, i32})  [unwired: 1 in]
                n782 = Decrement(x=w1812) -> (x-1=w1815:i32)
                n783 = Equal?(x=w1814, y=w1815) -> (x = y?=w1816:bool)
                n784 = case shown="False" w1816 {
                  tunnel: w1814 -> [w1947 _]
                  tunnel: [w1946 0] -> w1813
                  frame False {
                    n785 = Increment(x=w1947) -> (x+1=w1946:i32)
                  }
                  frame True {
                  }
                }
                n786 = Index Array(array=w1817, index=w1813) -> (element=w1818:string)
                n787 = local write "Data Name"(w1818) -> ()
                n788 = Concatenate Strings(w1825, "\\", w1818) -> (w1823:string)
                n789 = property on="Image Out" class="ImageControl"(error in=w1746, "Image Center Position"=w1749) -> ()  [unwired: 1 in, 2 out]
                n790 = String To Path(string=w1823) -> (path=w1773:path)
                n791 = call "sub_thresh_swing_subvi.vi"("Path"=w1773, "NumPts"=w1765, "Row Start"=w1771) -> ("Index"=w1766:dbl, "XY Graph"=w1761:cluster{dbl[], dbl[]}[], "Sub Threshold Swing"=w1774:dbl)  [unwired: 8 in, 2 out]
                n792 = Decimate 1D Array(w1761) -> (w1764:cluster{dbl[], dbl[]}[])  [unwired: 1 out]
                n793 = Array To Cluster(array=w1764) -> (cluster=w1762:T5)
                n794 = Unbundle(w1762) -> ("[0]"=w1763:cluster{dbl[], dbl[]})  [unwired: 8 out]
                n795 = Unbundle(w1763) -> (w1760:dbl[], w1759:dbl[])
                n796 = local write "S.T.S."(w1774) -> ()
                n797 = local write "XY Graph 2"(w1761) -> ()
                n798 = local write "Index 2"(w1766) -> ()
                n799 = call "mobility_subvi.vi"("Path"=w1773, "NumPts"=w1772, "Row Start"=w1771) -> ("Dielectric (d)"=w1777:dbl, "Index"=w1782:dbl, "XY Graph"=w1785:cluster{dbl[], dbl[]}[], "Length"=w1775:dbl, "Vt"=w1778:dbl, "Width"=w1776:dbl, "Table Control"=w1821:string[][], "Table Control 2"=w1820:string[][], "Recorded"=w1758:T6, "Mobility"=w1819:dbl)  [unwired: 2 in, 1 out]
                n800 = local write "Dielectric (d)"(w1777) -> ()
                n801 = local write "Threshold V"(w1778) -> ()
                n802 = local write "New Dielectric"(w1777) -> ()
                n803 = Decimate 1D Array(w1785) -> (w1786:cluster{dbl[], dbl[]}[])  [unwired: 1 out]
                n804 = Array To Cluster(array=w1786) -> (cluster=w1788:T5)
                n805 = local write "Table Control"(w1821) -> ()
                n806 = Unbundle(w1788) -> ("[0]"=w1787:cluster{dbl[], dbl[]})  [unwired: 8 out]
                n807 = Unbundle(w1787) -> (w1768:dbl[], w1767:dbl[])
                n808 = local write "XY Graph"(w1785) -> ()
                n809 = local write "Table Control 2"(w1820) -> ()
                n810 = local write "Mobility"(w1819) -> ()
                n811 = Array Subset(array=w1768, index=w1782, length=w1772) -> (w1784:dbl[])
                n812 = Array Subset(array=w1767, index=w1782, length=w1772) -> (w1783:dbl[])
                n813 = local write "Width"(w1776) -> ()
                n814 = local write "Length"(w1775) -> ()
                n815 = local write "Array 2"(w1783) -> ()
                n816 = Unbundle(w1758) -> ("Vt"=w1757:dbl, "STS"=w1756:dbl, "On/Off"=w1755:dbl)  [unwired: 4 out]
                n817 = local write "On/Off"(w1755) -> ()
                n818 = local write "Array"(w1784) -> ()
                n819 = local write "Slide"(w1782) -> ()
                n820 = local write "Index"(w1782) -> ()
                n821 = local write "STS recorded"(w1756) -> ()
                n822 = local write "Vt recorded"(w1757) -> ()
                n823 = Array Subset(array=w1760, index=w1766, length=w1765) -> (w1770:dbl[])
                n824 = Array Subset(array=w1759, index=w1766, length=w1765) -> (w1769:dbl[])
                n825 = local write "New Width"(w1776) -> ()
                n826 = local write "Data File"(w1773) -> ()
                n827 = local write "New Length"(w1775) -> ()
                n828 = local write "Array 8"(w1770) -> ()
                n829 = local write "Array 7"(w1769) -> ()
                n830 = call-poly <vilib>:"Read From Spreadsheet File.vi"("file path (dialog if empty)"=w1773) -> ("all rows"=w1808:string[][])  [unwired: 6 in, 4 out]
                n831 = local read "Image Folder"() -> (w1796:path)
                n832 = Array Size(array=w1808) -> (size(s)=w1807:i32[])
                n833 = List Folder(path=w1796) -> (filenames=w1801:string[])  [unwired: 3 in, 3 out]
                n834 = Index Array(array=w1807, index=w1806) -> (element=w1780:i32)
                n835 = Subtract(x=w1780, y=20) -> (x-y=w1779:i32)
                n836 = property on="Slide" class="Slide (strict)"("Scale.Maximum"=w1779) -> ()  [unwired: 2 in, 2 out]
                n837 = Array Subset(array=w1808, index (row)=w1806, index (col)=w1806, length (col)=3) -> (w1809:string[][])  [unwired: 1 in]
                n838 = Reshape Array(w1809, w1780) -> (w1789:string[])
                n839 = Search 1D Array(1D array=w1789, element="Mobility (cm^2/Vs):") -> (index of element=w1794:i32)  [unwired: 1 in]
                n840 = Search 1D Array(1D array=w1789, element="Index:") -> (index of element=w1803:i32)  [unwired: 1 in]
                n841 = Increment(x=w1803) -> (x+1=w1804:i32)
                n842 = Index Array(array=w1789, index=w1804) -> (element=w1799:string)
                n843 = while {
                  tunnel: w1801 -> [w1833]
                  tunnel: w1799 -> [w1831]
                  tunnel: [w1830] -> _
                  tunnel: [w1830] -> w1800
                  tunnel: w1780 -> [w1829]
                  i -> [w1830]
                  stop <- w1826 stop-if-true
                  n844 = Index Array(array=w1833, index=w1830) -> (element=w1834:string)
                  n845 = xnode "Match Regular Expression"("input string"=w1834, "regular expression"=w1831) -> ("whole match"=w1832:string)  [unwired: 4 in, 4 out]
                  n846 = Equal?(x=w1832, y=w1831) -> (x = y?=w1828:bool)
                  n847 = Equal?(x=w1829, y=w1830) -> (x = y?=w1827:bool)
                  n848 = Or(x=w1828, y=w1827) -> (x .or. y?=w1826:bool)
                }
                n849 = local write "Index 3"(w1799) -> ()
                n850 = Increment(x=w1794) -> (x+1=w1793:i32)
                n851 = local read "No Image"() -> (w1751:path)
                n852 = Index Array(array=w1789, index=w1793) -> (element=w1791:string)
                n853 = Fract/Exp String To Number(string=w1791) -> (number=w1790:dbl)  [unwired: 3 in, 1 out]
                n854 = local write "Recorded Mobility"(w1790) -> ()
                n855 = Path To String(path=w1796) -> (string=w1798:string)
                n856 = local read "Image Out"() -> (w1743:T2)
                n857 = Index Array(array=w1801, index=w1800) -> (element=w1753:string)
                n858 = Empty String/Path?(string/path=w1753) -> (empty?=w1754:bool)
                n859 = Concatenate Strings(w1798, "\\", w1753) -> (w1797:string)
                n860 = local write "Image Name"(w1753) -> ()
                n861 = String To Path(string=w1797) -> (path=w1752:path)
                n862 = Select(t=w1751, s=w1754, f=w1752) -> (s? t:f=w1745:path)
                n863 = local write "Image File"(w1745) -> ()
                n864 = call "IMAQ ReadFile"("File Path"=w1745, "Image"=w1743) -> ("Image Out"=w1744:T2)  [unwired: 5 in, 4 out]
                n865 = local write "Image Out 2"(w1744) -> ()
                n866 = local write "Image Out"(w1744) -> ()
                n867 = invoke on="Image Out" class="ImageControl" method="Clear ROI"() -> ()  [unwired: 3 in, 3 out]
              }
              frame #4 {
                n868 = local read "Image Folder"() -> (w1949:path)
                n869 = Build Path(base path=w1949, name or relative path="ROI") -> (appended path=w1951:path)
                n870 = local read "Index 3"() -> (w1950:string)
                n871 = Build Path(base path=w1951, name or relative path=w1950) -> (appended path=w1956:path)
                n872 = invoke on="Image Out" class="ImageControl" method="Clear ROI"() -> (error out=w1955:errorcluster)  [unwired: 3 in, 2 out]
                n873 = call <vilib>:"Check if File or Folder Exists.vi"("error in (no error)"=w1955, "path"=w1956) -> ("file or folder exists?"=w1953:bool, "dup path"=w1954:path)  [unwired: 7 in, 1 out]
                n874 = case shown="True" w1953 {
                  tunnel: w1954 -> [_ w1957]
                  frame False {
                  }
                  frame True {
                    n875 = Read from Text File(file (use dialog)=w1957) -> (text=w1961:string)  [unwired: 3 in, 3 out]
                    n876 = property on="Image Out" class="ImageControl"() -> ("ROI"=w1958:T7)  [unwired: 2 in, 2 out]
                    n877 = Unflatten From String(type=w1958, binary string=w1961) -> (value=w1959:T7, error out=w1960:errorcluster)  [unwired: 3 in, 1 out]
                    n878 = property on="Image Out" class="ImageControl"(error in=w1960, "ROI"=w1959) -> ()  [unwired: 1 in, 2 out]
                  }
                }
              }
            }
          }
          event "Export": Mouse Down {
            n879 = event-data() -> ()  [unwired: 1 in, 7 out]
            n880 = local read "Data Folder"() -> (w1962:path)
            n881 = call "OA_ConnectToOrigin.vi"() -> ("error out"=w1983:errorcluster, "Origin.IOApplication"=w1984:refnum<k7>)  [unwired: 8 in]
            n882 = local read "Project"() -> (w1982:path)
            n883 = call "OA_Load.vi"("error in (no error)"=w1983, "Path"=w1982, "Origin.IOApplication"=w1984) -> ("error out"=w1975:errorcluster, "Origin.IOApplication"=w1976:refnum<k7>)  [unwired: 1 out]
            n884 = call "OAExecute.vi"("script"="document -m 3;", "Error IO"=w1975, "Origin.IOApplication"=w1976) -> ("Error IO Out"=w1973:errorcluster, "Origin.IOApplication"=w1974:refnum<k7>)  [unwired: 1 in, 1 out]
            n885 = Build Path(base path=w1962, name or relative path="Stats") -> (appended path=w1963:path)
            n886 = flat-sequence {
              tunnel: w1962 -> [w2004]
              tunnel: w1981 -> [w2003]
              tunnel: [w1993] -> w1986
              tunnel: [w1994] -> w1985
              tunnel: w1974 -> [w1998]
              tunnel: w1973 -> [w1997]
              tunnel: w1962 -> [w2020]
              tunnel: w1981 -> [w2019]
              tunnel: w1986 -> [w2015]
              tunnel: w1985 -> [w2016]
              tunnel: [w2010] -> w1980
              tunnel: [w2009] -> w1979
              tunnel: w1962 -> [w2031]
              tunnel: w1981 -> [w2030]
              tunnel: w1980 -> [w2026]
              tunnel: w1979 -> [w2025]
              tunnel: [w2024] -> w1978
              tunnel: [w2023] -> w1977
              tunnel: w1962 -> [w2046]
              tunnel: w1981 -> [w2045]
              tunnel: w1978 -> [w2040]
              tunnel: w1977 -> [w2039]
              tunnel: [w2037] -> w1971
              tunnel: [w2036] -> w1970
              frame #0 {
                n887 = call "Param_Analysis.vi"("error in (no error)"=w1997, "Folder 2"=w2004, "Parameter String"="Mobility (cm^2/Vs):", "Parameter Name"="Mobility", "Folder"=w2003) -> ("error out"=w2000:errorcluster, "Array 4"=w1990:string[], "Array 3"=w1999:string[][])  [unwired: 3 in, 1 out]
                n888 = call "Origin_Export.vi"("String 3"="[MobHistTab]Sheet1", "error in (no error)"=w2000, "Array"=w1999, "String 2"="[MOBvsLTable]Mobilities", "String"="pe_cd \"Mobility Chart\";", "Origin.IOApplication"=w1998, "Array 2"=w1990) -> ("reference out"=w1996:refnum<k7>, "error out"=w1995:errorcluster)  [unwired: 2 in, 1 out]
                n889 = call "OAExecute.vi"("script"="window -a MOBvsLTable;\nwindow -s TV;", "Error IO"=w1995, "Origin.IOApplication"=w1996) -> ("Error IO Out"=w1993:errorcluster, "Origin.IOApplication"=w1994:refnum<k7>)  [unwired: 1 in, 1 out]
              }
              frame #1 {
                n890 = call "Param_Analysis.vi"("error in (no error)"=w2015, "Folder 2"=w2020, "Parameter String"="On/Off Current:", "Parameter Name"="On_Off_Current", "Folder"=w2019) -> ("error out"=w2014:errorcluster, "Array 4"=w2008:string[], "Array 3"=w2011:string[][])  [unwired: 3 in, 1 out]
                n891 = call "Origin_Export.vi"("String 3"="[OnOffHistTab]Sheet1", "error in (no error)"=w2014, "Array"=w2011, "String 2"="[OnOffTable]On/Off Ratios", "String"="pe_cd \"OnOff vs L\";", "Origin.IOApplication"=w2016, "Array 2"=w2008) -> ("reference out"=w2010:refnum<k7>, "error out"=w2009:errorcluster)  [unwired: 2 in, 1 out]
              }
              frame #2 {
                n892 = call "Param_Analysis.vi"("Folder 2"=w2031, "Parameter String"="S.T.S. (V/decade):", "Parameter Name"="STS", "Folder"=w2030) -> ("Array 4"=w2022:string[], "Array 3"=w2027:string[][])  [unwired: 4 in, 2 out]
                n893 = call "Origin_Export.vi"("String 3"="[SHistTab]Sheet1", "error in (no error)"=w2025, "Array"=w2027, "String 2"="[STable]Threshold Swing", "String"="pe_cd \"Threshold Swing vs L\";", "Origin.IOApplication"=w2026, "Array 2"=w2022) -> ("reference out"=w2023:refnum<k7>, "error out"=w2024:errorcluster)  [unwired: 2 in, 1 out]
              }
              frame #3 {
                n894 = call "Param_Analysis.vi"("Folder 2"=w2046, "Parameter String"="Threshold V (V):", "Parameter Name"="Threshold_V", "Folder"=w2045) -> ("Array 4"=w2035:string[], "Array 3"=w2038:string[][])  [unwired: 4 in, 2 out]
                n895 = call "Origin_Export.vi"("String 3"="[VtHistTab]Sheet1", "error in (no error)"=w2040, "Array"=w2038, "String 2"="[VtTable]Threshold Voltages", "String"="pe_cd \"Threshold Voltage vs L\";", "Origin.IOApplication"=w2039, "Array 2"=w2035) -> ("reference out"=w2037:refnum<k7>, "error out"=w2036:errorcluster)  [unwired: 2 in, 1 out]
              }
            }
            n896 = call <vilib>:"Check if File or Folder Exists.vi"("path"=w1963) -> ("file or folder exists?"=w1988:bool, "dup path"=w1987:path)  [unwired: 8 in, 1 out]
            n897 = case shown="False" w1988 {
              tunnel: w1987 -> [w2048 w2049]
              tunnel: [w2047 w2049] -> w1981
              frame False {
                n898 = Create Folder(path (use dialog)=w2048) -> (created path=w2047:path)  [unwired: 2 in, 2 out]
              }
              frame True {
              }
            }
            n899 = call "File Dialog"("start path"=w1963) -> ("selected path"=w1966:path)  [unwired: 11 in, 3 out]
            n900 = Path To String(path=w1966) -> (string=w1965:string)
            n901 = call "OAExecute.vi"("script"="pe_cd /;\npe_cd \"Mobility Chart\"; ", "Error IO"=w1970, "Origin.IOApplication"=w1971) -> ("Error IO Out"=w1967:errorcluster, "Origin.IOApplication"=w1968:refnum<k7>)  [unwired: 1 in, 1 out]
            n902 = call "OASaveProject.vi"("path"=w1965, "Error IO"=w1967, "Origin.IOApplication"=w1968) -> ()  [unwired: 3 out]
          }
          event "Blank Button": Mouse Down {
            n903 = event-data() -> ()  [unwired: 1 in, 7 out]
            n904 = local read "Data File"() -> (w2057:path)
            n905 = Strip Path(path=w2057) -> (stripped path=w2053:path, name=w2055:string)
            n906 = Path To String(path=w2053) -> (string=w2052:string)
            n907 = Concatenate Strings(w2052, "\\", "X_", w2055) -> (w2051:string)
            n908 = String To Path(string=w2051) -> (path=w2050:path)
            n909 = Move(source path=w2057, 10:w2050) -> ()  [unwired: 3 in, 3 out]
            n910 = local write "Data File"(w2050) -> ()
          }
          event "Cancel Button": Mouse Down {
            (unwired) 6
            n911 = event-data() -> ()  [unwired: 1 in, 7 out]
            n912 = call "Simulate_Keyboard.vi"("Action"=2, "Virtual Key"=162) -> ()  [unwired: 7 in, 1 out]
          }
        }
        n913 = property on="Image Out" class="ImageControl"() -> ("ROI"=w366:T7)  [unwired: 2 in, 2 out]
        n914 = local read "Image Out"() -> (w395:T2)
        n915 = property on="Image Out" class="ImageControl"() -> ("ZoomSingle"=w409:cluster{"X":sgl, "Y":sgl})  [unwired: 2 in, 2 out]
        n916 = property on="Image Out" class="ImageControl"() -> ("Bounds"=w410:T8)  [unwired: 2 in, 2 out]
        n917 = Unbundle By Name(w366) -> ("Contours"=w440:T9)
        n918 = call <vilib>:"Intialize Keyboard.vi"() -> ("device ID"=w421:refnum<k1>)  [unwired: 10 in, 1 out]
        n919 = property on="Image Out" class="ImageControl"() -> ("Image Center Position"=w416:cluster{"X":u32, "Y":u32})  [unwired: 2 in, 2 out]
        n920 = call "IMAQ Clear Overlay"("Image"=w395) -> ("Image Out"=w394:T2)  [unwired: 9 in, 1 out]
        n921 = call-poly <vilib>:"Acquire Input Data.vi"("device ID"=w421) -> ("keys pressed"=w420:T10)  [unwired: 16 in, 2 out]
        n922 = Initialize Array(0) -> (w438:i32[])  [unwired: 1 in]
        n923 = local read "Magnification"() -> (w429:u16)
        n924 = Unbundle(w410) -> ("Width"=w407:u32, "Height"=w406:u32)
        n925 = Array Size(array=w440) -> (size(s)=w439:i32)
        n926 = Unbundle(w409) -> ("X"=w384:sgl, "Y"=w408:sgl)
        n927 = event shown="[2] \" Image Folder\": Value Change" {
          selector: _ -> [_ _ _ _ _ _ _]
          dyn-events: _ -> [_ _ _ _ _ _ _]
          timeout: 10 -> [_ _ _ _ _ _ _]
          event "Remove Button": Mouse Down {
            w446 = 0
            n928 = property on="Image Out" class="ImageControl"() -> ("ROI"=w444:T7)  [unwired: 2 in, 2 out]
            n929 = event-data() -> ()  [unwired: 1 in, 7 out]
            n930 = Unbundle(w444) -> ("Global Rectangle"=w447:i32[], "Contours"=w449:T9)
            n931 = Reverse 1D Array(array=w447) -> (reversed array=w448:i32[])
            n932 = Reverse 1D Array(array=w449) -> (reversed array=w450:T9)
            n933 = Delete From Array(array=w448, index=w446) -> (array with subset deleted=w451:i32[])  [unwired: 1 in, 1 out]
            n934 = Delete From Array(array=w450, index=w446) -> (array with subset deleted=w452:T9)  [unwired: 1 in, 1 out]
            n935 = Reverse 1D Array(array=w451) -> (reversed array=w453:i32[])
            n936 = Reverse 1D Array(array=w452) -> (reversed array=w454:T9)
            n937 = Bundle(w453, w454) -> (w445:T11)  [unwired: 1 in]
            n938 = local write "ROI Descriptor out"(w444) -> ()
            n939 = local write "ROI Descriptor"(w445) -> ()
            n940 = property on="Image Out" class="ImageControl"("ROI"=w445) -> ()  [unwired: 2 in, 2 out]
          }
          event "Undo Button": Mouse Down {
            n941 = event-data() -> ()  [unwired: 1 in, 7 out]
            n942 = invoke on="Image Out" class="ImageControl" method="Clear ROI"() -> ()  [unwired: 3 in, 3 out]
          }
          event "Image Folder": Value Change {
            n943 = event-data() -> ()  [unwired: 1 in, 5 out]
            n944 = local read "Image File"() -> (w456:path)
            n945 = call "Vision Acquisition"("Image Path"=w456) -> ("Image Out"=w455:T2)  [unwired: 25 in, 1 out]
            n946 = local write "Image Out 2"(w455) -> ()
            n947 = local write "Image Out"(w455) -> ()
            n948 = invoke on="Image Out" class="ImageControl" method="Clear ROI"() -> ()  [unwired: 3 in, 3 out]
          }
          event "Zoom": Value Change {
            n949 = event-data() -> ()  [unwired: 1 in, 5 out]
            n950 = local read "Zoom"() -> (w457:i16)
            n951 = Bundle("Zoom"=w457, "Zoom"=w457) -> (w458:cluster{"Zoom":i16, "Zoom":i16})  [unwired: 1 in]
            n952 = property on="Image Out" class="ImageControl"("ZoomInteger"=w458) -> ()  [unwired: 2 in, 2 out]
          }
          event Timeout {
            n953 = event-data() -> ()  [unwired: 1 in, 2 out]
          }
          event "Image Out": Mouse Enter {
            (unwired) 6
            n954 = event-data() -> ()  [unwired: 1 in, 3 out]
            n955 = call "Simulate_Keyboard.vi"("Action"=0, "Virtual Key"=162) -> ()  [unwired: 7 in, 1 out]
          }
          event "Image Out": Mouse Leave {
            n956 = event-data() -> ()  [unwired: 1 in, 3 out]
            n957 = flat-sequence {
              frame #0 {
                n958 = Wait (ms)(milliseconds to wait=10) -> ()  [unwired: 1 out]
              }
              frame #1 {
                (unwired) 6
                n959 = call "Simulate_Keyboard.vi"("Action"=2, "Virtual Key"=162) -> ()  [unwired: 7 in, 1 out]
              }
            }
          }
        }
        n960 = Build Array(0.505025, 0.252522, 0.127742, 0.050345, 0.031129) -> (w430:dbl[])
        n961 = Index Array(array=w420) -> (element=w424:T12)  [unwired: 1 in]
        n962 = Divide(x=w407, y=w384) -> (x/y=w397:sgl)
        n963 = Multiply(x=w397, y=0.5) -> (x*y=w403:dbl)
        n964 = Divide(x=w406, y=w408) -> (x/y=w396:sgl)
        n965 = Multiply(x=w396, y=0.5) -> (x*y=w402:dbl)
        n966 = Array Subset(array=w430, index=w429, length=1) -> (w427:dbl[])
        n967 = property on="Image Out" class="ImageControl"() -> ("ZoomInteger"=w419:cluster{"X":i32, "Y":i32})  [unwired: 2 in, 2 out]
        n968 = Unbundle(w416) -> ("X"=w398:u32, "Y"=w399:u32)
        n969 = Subtract(x=w399, y=w402) -> (x-y=w400:dbl)
        n970 = Subtract(x=w398, y=w403) -> (x-y=w401:dbl)
        n971 = Add(x=w401, y=w397) -> (x+y=w415:dbl)
        n972 = Add(x=w400, y=w396) -> (x+y=w414:dbl)
        n973 = To Double Precision Float(number=w427) -> (double precision float=w426:dbl[])
        n974 = local write "ROI Descriptor"(w366) -> ()
        n975 = Reciprocal(x=w384) -> (1/x=w383:sgl)
        n976 = Unbundle(w419) -> ("X"=w418:i32)  [unwired: 1 out]
        n977 = Multiply(x=w383, y=10) -> (x*y=w385:sgl)
        n978 = case shown="\"EQUALS\"" w424 {
          tunnel: w398 -> [w465 w471 w475 w477 w481 w483 w485 w487 w489 w491 w493 w495 w497 w499 w501 w503 w505 w507 w509 w511 w513 w515 w517 w519 w521 w523 w525 w527 w529 w531 w533 w535 w537 w539 w541 w543 w545 w547 w549 w551 w553 w555 w557 w559 w561 w563 w565 w567 w569 w571 w573 w575 w577 w579 w581 w583 w585 w587 w589 w591 w593 w595 w597 w599 w601 w603 w605 w607 w609 w611 w613 w615 w617 w619 w621 w623 w625 w627 w629 w631 w633 w635 w637 w639 w641 w643 w645 w647 w649 w651 w653 w655 w657 w659 w661 w663 w665 w667 w669 w671 w673 w675 w677 w679 w681]
          tunnel: [w465 w470 w474 w477 w481 w483 w485 w487 w489 w491 w493 w495 w497 w499 w501 w503 w505 w507 w509 w511 w513 w515 w517 w519 w521 w523 w525 w527 w529 w531 w533 w535 w537 w539 w541 w543 w545 w547 w549 w551 w553 w555 w557 w559 w561 w563 w565 w567 w569 w571 w573 w575 w577 w579 w581 w583 w585 w587 w589 w591 w593 w595 w597 w599 w601 w603 w605 w607 w609 w611 w613 w615 w617 w619 w621 w623 w625 w627 w629 w631 w633 w635 w637 w639 w641 w643 w645 w647 w649 w651 w653 w655 w657 w659 w661 w663 w665 w667 w669 w671 w673 w675 w677 w679 w681] -> w423
          tunnel: w399 -> [w467 w469 w473 w479 w480 w482 w484 w486 w488 w490 w492 w494 w496 w498 w500 w502 w504 w506 w508 w510 w512 w514 w516 w518 w520 w522 w524 w526 w528 w530 w532 w534 w536 w538 w540 w542 w544 w546 w548 w550 w552 w554 w556 w558 w560 w562 w564 w566 w568 w570 w572 w574 w576 w578 w580 w582 w584 w586 w588 w590 w592 w594 w596 w598 w600 w602 w604 w606 w608 w610 w612 w614 w616 w618 w620 w622 w624 w626 w628 w630 w632 w634 w636 w638 w640 w642 w644 w646 w648 w650 w652 w654 w656 w658 w660 w662 w664 w666 w668 w670 w672 w674 w676 w678 w680]
          tunnel: [w466 w469 w473 w478 w480 w482 w484 w486 w488 w490 w492 w494 w496 w498 w500 w502 w504 w506 w508 w510 w512 w514 w516 w518 w520 w522 w524 w526 w528 w530 w532 w534 w536 w538 w540 w542 w544 w546 w548 w550 w552 w554 w556 w558 w560 w562 w564 w566 w568 w570 w572 w574 w576 w578 w580 w582 w584 w586 w588 w590 w592 w594 w596 w598 w600 w602 w604 w606 w608 w610 w612 w614 w616 w618 w620 w622 w624 w626 w628 w630 w632 w634 w636 w638 w640 w642 w644 w646 w648 w650 w652 w654 w656 w658 w660 w662 w664 w666 w668 w670 w672 w674 w676 w678 w680] -> w422
          tunnel: w385 -> [w464 w468 w472 w476 _ _ _ _ _ _ _ _ _ _ _ _ _ _ _ _ _ _ _ _ _ _ _ _ _ _ _ _ _ _ _ _ _ _ _ _ _ _ _ _ _ _ _ _ _ _ _ _ _ _ _ _ _ _ _ _ _ _ _ _ _ _ _ _ _ _ _ _ _ _ _ _ _ _ _ _ _ _ _ _ _ _ _ _ _ _ _ _ _ _ _ _ _ _ _ _ _ _ _ _ _]
          frame "DOWN" {
            n979 = Add(x=w467, y=w464) -> (x+y=w466:sgl)
          }
          frame "LEFT" {
            n980 = Subtract(x=w471, y=w468) -> (x-y=w470:sgl)
          }
          frame "RIGHT" {
            n981 = Add(x=w475, y=w472) -> (x+y=w474:sgl)
          }
          frame "UP" {
            n982 = Subtract(x=w479, y=w476) -> (x-y=w478:sgl)
          }
          frame "ENTER (num pad)" {
          }
          frame "' (quote)" {
          }
          frame "END" {
          }
          frame "EQUALS" {
          }
          frame "ESCAPE" {
          }
          frame "GRAVE (`)" {
          }
          frame "HOME" {
          }
          frame "INSERT" {
          }
          frame "LBRACKET" {
          }
          frame "LCONTROL" {
          }
          frame "L ALT" {
          }
          frame "LSHIFT" {
          }
          frame "LWIN" {
          }
          frame "MINUS" {
          }
          frame "MULTIPLY" {
          }
          frame "NEXT" {
          }
          frame "NUMLOCK" {
          }
          frame "NUMPAD_0" {
          }
          frame "NUMPAD_1" {
          }
          frame "NUMPAD_2" {
          }
          frame "NUMPAD_3" {
          }
          frame "NUMPAD_4" {
          }
          frame "NUMPAD_5" {
          }
          frame "NUMPAD_6" {
          }
          frame "NUMPAD_7" {
          }
          frame "NUMPAD_8" {
          }
          frame "NUMPAD_9" {
          }
          frame "PAUSE" {
          }
          frame "PERIOD" {
          }
          frame "PRIOR (PG UP)" {
          }
          frame "RBRACKET" {
          }
          frame "RCONTROL" {
          }
          frame "RETURN" {
          }
          frame "R ALT" {
          }
          frame "RSHIFT" {
          }
          frame "RWIN" {
          }
          frame "SCROLL" {
          }
          frame "SEMICOLON" {
          }
          frame "SLASH" {
          }
          frame "SPACE" {
          }
          frame "SUBTRACT" {
          }
          frame "TAB" {
          }
          frame "DIVIDE" {
          }
          frame "DELETE" {
          }
          frame "DECIMAL" {
          }
          frame "COMMA" {
          }
          frame "CAPITAL" {
          }
          frame "BACKSLASH" {
          }
          frame "BACK" {
          }
          frame "ADD" {
          }
          frame "F15" {
          }
          frame "F14" {
          }
          frame "F13" {
          }
          frame "F12" {
          }
          frame "F11" {
          }
          frame "F10" {
          }
          frame "F9" {
          }
          frame "F8" {
          }
          frame "F7" {
          }
          frame "F6" {
          }
          frame "F5" {
          }
          frame "F4" {
          }
          frame "F3" {
          }
          frame "F2" {
          }
          frame "F1" {
          }
          frame "Z" {
          }
          frame "Y" {
          }
          frame "X" {
          }
          frame "W" {
          }
          frame "V" {
          }
          frame "U" {
          }
          frame "T" {
          }
          frame "S" {
          }
          frame "R" {
          }
          frame "Q" {
          }
          frame "P" {
          }
          frame "O" {
          }
          frame "N" {
          }
          frame "M" {
          }
          frame "L" {
          }
          frame "K" {
          }
          frame "J" {
          }
          frame "I" {
          }
          frame "H" {
          }
          frame "G" {
          }
          frame "F" {
          }
          frame "E" {
          }
          frame "D" {
          }
          frame "C" {
          }
          frame "B" {
          }
          frame "A" {
          }
          frame "9" {
          }
          frame "8" {
          }
          frame "7" {
          }
          frame "6" {
          }
          frame "5" {
          }
          frame "4" {
          }
          frame "3" {
          }
          frame "2" {
          }
          frame "1" {
          }
          frame "0" {
          }
        }
        n983 = Bundle(w401, w400, w415, w414, 0.0) -> (w413:cluster{dbl, dbl, dbl, dbl, dbl})  [unwired: 1 in]
        n984 = Bundle("X"=w423, "Y"=w422) -> (w417:cluster{"X":sgl, "Y":sgl})  [unwired: 1 in]
        n985 = Divide(x=20, y=w384) -> (x/y=w387:sgl)
        n986 = local write "Zoom"(w418) -> ()
        n987 = property on="Image Out" class="ImageControl"("Image Center Position"=w417) -> ()  [unwired: 2 in, 2 out]
        n988 = call "IMAQ Convert Rectangle to ROI (Polygon)"("Rectangle"=w413) -> ("ROI Descriptor"=w411:T3)  [unwired: 7 in, 2 out]
        n989 = Bundle("Application Font", w387, w391, w391, w391, w391, w391, TRUE, w389) -> (w393:T13)  [unwired: 1 in]
        n990 = property on="Image Out 2" class="ImageControl"("ROI"=w411) -> ()  [unwired: 2 in, 2 out]
        n991 = Bundle(w389, w393, w389, w389) -> (w392:T14)  [unwired: 1 in]
        n992 = for {
          N: w439 -> [_]
          shift-right: [w704] -> _
          shift-left: w440 -> [w704]
          shift-right: [w702] -> w425
          shift-left: w438 -> [w701]
          tunnel: w426 -> [w700]
          shift-right: [w697] -> _
          shift-left: w394 -> [w699]
          tunnel: w392 -> [w692]
          i -> [w696]
          n993 = Index Array(array=w704, index=w696) -> (element=w713:T15)
          n994 = Unbundle(w713) -> ("Points"=w712:i32[])  [unwired: 2 out]
          n995 = Array To Cluster(array=w712) -> (cluster=w711:T16)
          n996 = Unbundle(w711) -> ("Points[0]"=w691:i32, "Points[1]"=w688:i32, "Points[2]"=w703:i32, "Points[3]"=w709:i32)  [unwired: 5 out]
          n997 = Add(x=w691, y=10) -> (x+y=w689:i32)
          n998 = Subtract(x=w688, y=w709) -> (x-y=w708:i32)
          n999 = Subtract(x=w691, y=w703) -> (x-y=w710:i32)
          n1000 = Square(x=w708) -> (x^2=w706:i32)
          n1001 = Square(x=w710) -> (x^2=w707:i32)
          n1002 = Add(x=w707, y=w706) -> (x+y=w705:i32)
          n1003 = Square Root(x=w705) -> (sqrt(x)=w682:dbl)
          n1004 = Multiply(x=w682, y=0.5) -> (x*y=w685:dbl)
          n1005 = Add(x=w685, y=w688) -> (x+y=w687:dbl)
          n1006 = Bundle(w689, w687) -> (w698:cluster{i32, dbl})  [unwired: 1 in]
          n1007 = Multiply(x=w682, y=w700) -> (x*y=w695:dbl[])
          n1008 = Index Array(array=w695) -> (element=w694:dbl)  [unwired: 1 in]
          n1009 = Number To Fractional String(number=w694) -> (F-format string=w693:string)  [unwired: 3 in]
          n1010 = call "IMAQ Overlay Text"("BG Color (Transparent)"=u32 0, "Text Color (black)"=u32 16448250, "Font, Size & Style"=w692, "String"=w693, "Origin"=w698, "Image"=w699) -> ("Image Out"=w697:T2)  [unwired: 4 in, 1 out]
          n1011 = Build Array (concatenate)(w701, w695) -> (w702:dbl[])
          n1012 = local write "Numeric 3"(w682) -> ()
        }
        n1013 = Add Array Elements(numeric array=w425) -> (sum=w436:dbl)
        n1014 = local write "Distances"(w425) -> ()
        n1015 = local write "Total Width"(w436) -> ()
        n1016 = local read "Array 8"() -> (w371:dbl[])
        n1017 = local read "Array 7"() -> (w372:dbl[])
        n1018 = local read "Width"() -> (w367:dbl)
        n1019 = local read "New Dielectric"() -> (w379:dbl)
        n1020 = local read "Array 2"() -> (w375:dbl[])
        n1021 = local read "Manual"() -> (w365:bool)
        n1022 = local read "New Length"() -> (w377:dbl)
        n1023 = local read "Array"() -> (w376:dbl[])
        n1024 = call "sts_calc_subvi.vi"("Array 2"=w371, "Array"=w372) -> ("STS"=w373:dbl)  [unwired: 9 in]
        n1025 = local read "New Width"() -> (w380:dbl)
        n1026 = local write "New S.T.S."(w373) -> ()
        n1027 = call "mob_calc_subvi.vi"("Width"=w380, "Length"=w377, "Dielectric (d)"=w379, "Array 2"=w375, "Array"=w376) -> ("Vt"=w374:dbl, "Mobility"=w378:dbl)  [unwired: 5 in]
        n1028 = Not(x=w365) -> (.not. x?=w363:bool)
        n1029 = local write "New Vt"(w374) -> ()
        n1030 = local write "New Mobility"(w378) -> ()
        n1031 = local read "Total Width"() -> (w369:dbl)
        n1032 = Equal To 0?(x=w369) -> (x = 0?=w364:bool)
        n1033 = And(x=w364, y=w363) -> (x .and. y?=w362:bool)
        n1034 = case shown="True" w362 {
          tunnel: w367 -> [_ w442]
          frame False {
          }
          frame True {
            n1035 = local write "New Width"(w442) -> ()
          }
        }
        n1036 = Or(x=w364, y=w365) -> (x .or. y?=w368:bool)
        n1037 = case shown="False" w368 {
          tunnel: w369 -> [w443 _]
          frame False {
            n1038 = local write "New Width"(w443) -> ()
          }
          frame True {
          }
        }
      }
    }
  }
  n1039 = Divide(x="RPM:", y="Ramp (s):") -> (x/y=→"Accel (RPM/s):":dbl)
  n1040 = disable-structure shown="Disabled" {
    frame Disabled {
      n1041 = local read "Data Folder"() -> ()  [unwired: 1 out]
      n1042 = local read "Data Folder"() -> ()  [unwired: 1 out]
      n1043 = local read "Data Folder"() -> ()  [unwired: 1 out]
    }
    frame Enabled {
    }
  }
